vi "BRig_RT_panel_Laser1_v1,12.vi"(7 "input_setValues":bool, 9 "input_dataExp":u16[](array[numeric]), 11 "input_dataLC":u16[](array[numeric])) -> (1 "output_dataExp":u16[](array[numeric]), 3 "output_dataLC":u16[](array[numeric]))   [LabVIEW 2014]
panel:
  in  "LC_Wro_nRew2":u16
  in  "LC_Wro_nRew1":u16
  in  "LC_Rew_nRew2":u16
  in  "LC_Rew_nRew1":u16
  in  "LC_Sel_nRew2":u16
  in  "LC_Sel_nRew1":u16
  in  "LC_Cue2_nRew2":u16
  in  "LC_Cue2_nRew1":u16
  in  "LC_Cue_nRew2":u16
  in  "LC_Cue_nRew1":u16
  in  "LC_ENL2_nRew2":u16
  in  "LC_ENL2_nRew1":u16
  in  "LC_ENL_nRew2":u16
  in  "LC_ENL_nRew1":u16
  in  "LC_Cue2_PostR_Count":u16
  in  "LC_Cue2_PostR_delayOpt":bool
  in  "LC_Cue2_PostR_Probability":u16
  in  "LC_Cue2_PostR_Block":u16(slide) max=2 step=1 scale=0.0..2.0
  in  "LC_Cue2_PostR_OnOff":bool
  in  "LC_Cue2_PostR_Tdelay":u16
  in  "LC_ENL2_PostR_delayOpt":bool
  in  "LC_ENL2_PostR_Count":u16
  in  "LC_ENL2_PostR_Probability":u16 max=100 step=1
  in  "LC_ENL2_PostR_Block":u16(slide) max=2 step=1 scale=0.0..2.0
  in  "LC_ENL2_PostR_OnOff":bool
  in  "LC_ENL2_PostR_Tdelay":u16
  in  "LC_Cue2_PreR_Count":u16
  in  "LC_Cue2_First_Count":u16
  in  "LC_Cue2_PreR_delayOpt":bool
  in  "LC_ENL2_PreR_delayOpt":bool
  in  "LC_ENL2_PreR_Count":u16
  in  "LC_ENL2_First_Count":u16
  in  "LC_Cue2_First_delayOpt":bool
  in  "LC_ENL2_First_delayOpt":bool
  in  "LC_Cue2_PreR_Probability":u16
  in  "LC_Cue2_PreR_Block":u16(slide) max=2 step=1 scale=0.0..2.0
  in  "LC_Cue2_PreR_OnOff":bool
  in  "LC_Cue2_First_Probability":u16
  in  "LC_Cue2_First_Block":u16(slide) max=2 step=1 scale=0.0..2.0
  in  "LC_Cue2_First_OnOff":bool
  in  "LC_ENL2_PreR_Probability":u16 max=100 step=1
  in  "LC_ENL2_PreR_Block":u16(slide) max=2 step=1 scale=0.0..2.0
  in  "LC_ENL2_PreR_OnOff":bool
  in  "LC_ENL2_First_Probability":u16 max=100 step=1
  in  "LC_ENL2_First_Block":u16(slide) max=2 step=1 scale=0.0..2.0
  in  "LC_Cue2_PreR_Tdelay":u16
  in  "LC_ENL2_PreR_Tdelay":u16
  in  "LC_Cue2_First_Tdelay":u16
  in  "LC_ENL2_First_Tdelay":u16
  in  "LC_ENL2_First_OnOff":bool
  out "LaserPulseTrain":cluster{u16[], u16[]}(graph)
  in  "LED_baseline":bool
  in  "Laser_power_step":dbl
  in  "Laser_power_max":dbl
  in  "Laser_power_min":dbl
  in  "Laser_Tshutter":u16=2
  in  "Laser_Freq":u16=10
  in  "Laser_Tpeak":u16=2
  in  "Laser_T":u16
  in  "LC_Sel_PostR_Count":u16
  in  "LC_Sel_PostR_Probability":u16
  in  "LC_Sel_PostR_Block":u16(slide) max=2 step=1 scale=0.0..2.0
  in  "LC_Sel_PostR_OnOff":bool
  in  "LC_Sel_PostR_Tdelay":u16
  in  "LC_Cue_PostR_Count":u16
  in  "LC_Cue_PostR_delayOpt":bool
  in  "LC_Cue_PostR_Probability":u16
  in  "LC_Cue_PostR_Block":u16(slide) max=2 step=1 scale=0.0..2.0
  in  "LC_Cue_PostR_OnOff":bool
  in  "LC_Cue_PostR_Tdelay":u16
  in  "LC_ENL_PostR_delayOpt":bool
  in  "LC_ENL_PostR_Count":u16
  in  "LC_ENL_PostR_Probability":u16 max=100 step=1
  in  "LC_ENL_PostR_Block":u16(slide) max=2 step=1 scale=0.0..2.0
  in  "LC_ENL_PostR_OnOff":bool
  in  "LC_ENL_PostR_Tdelay":u16
  in  "LC_Sel_PreR_Count":u16
  in  "LC_Sel_First_Count":u16
  in  "LC_Sel_PreR_Probability":u16
  in  "LC_Sel_PreR_Block":u16(slide) max=2 step=1 scale=0.0..2.0
  in  "LC_Sel_PreR_OnOff":bool
  in  "LC_Sel_First_Probability":u16
  in  "LC_Sel_First_Block":u16(slide) max=2 step=1 scale=0.0..2.0
  in  "LC_Sel_First_OnOff":bool
  in  "LC_Sel_PreR_Tdelay":u16
  in  "LC_Sel_First_Tdelay":u16
  in  "LC_Cue_PreR_Count":u16
  in  "LC_Cue_First_Count":u16
  in  "LC_Cue_PreR_delayOpt":bool
  in  "LC_ENL_PreR_delayOpt":bool
  in  "LC_ENL_PreR_Count":u16
  in  "LC_ENL_First_Count":u16
  in  "LC_Cue_First_delayOpt":bool
  in  "LC_ENL_First_delayOpt":bool
  in  "LC_Wrong_Probability":u16
  in  "LC_Wrong_Trial":u16(slide) max=3 step=1 scale=0.0..3.0
  in  "LC_Wrong_Block":u16(slide) max=2 step=1 scale=0.0..2.0
  in  "LC_Wrong_OnOff":bool
  in  "LC_Reward_Probability":u16
  in  "LC_Reward_Trial":u16(slide) max=3 step=1 scale=0.0..3.0
  in  "LC_Reward_Block":u16(slide) max=2 step=1 scale=0.0..2.0
  in  "LC_Reward_OnOff":bool
  in  "LC_Cue_PreR_Probability":u16
  in  "LC_Cue_PreR_Block":u16(slide) max=2 step=1 scale=0.0..2.0
  in  "LC_Cue_PreR_OnOff":bool
  in  "LC_Cue_First_Probability":u16
  in  "LC_Cue_First_Block":u16(slide) max=2 step=1 scale=0.0..2.0
  in  "LC_Cue_First_OnOff":bool
  in  "LC_ENL_PreR_Probability":u16 max=100 step=1
  in  "LC_ENL_PreR_Block":u16(slide) max=2 step=1 scale=0.0..2.0
  in  "LC_ENL_PreR_OnOff":bool
  in  "LC_ENL_First_Probability":u16 max=100 step=1
  in  "LC_ENL_First_Block":u16(slide) max=2 step=1 scale=0.0..2.0
  in  "LC_Wrong_Tdelay":u16
  in  "LC_Cue_PreR_Tdelay":u16
  in  "LC_ENL_PreR_Tdelay":u16
  in  "LC_Reward_Tdelay":u16
  in  "LC_Cue_First_Tdelay":u16
  in  "LC_ENL_First_Tdelay":u16
  in  "LC_ENL_First_OnOff":bool
  # "Laser1 Control\n                               On/Off      Block        Probability [%]   Delay [ms]                              Count"
  # "On/Off      Block        Probability [%]   Delay [ms]                              Count"
  # "Enforced\nNonLick"
  # "Enforced\nNonLick\n     2"
  # "from end"
  # "from end"
  # "First\nTrial"
  # "First\nTrial"
  # "from start"
  # "from start"
  # "from end"
  # "from end"
  # "PreReward\nTrials"
  # "PreReward\nTrials"
  # "from start"
  # "from start"
  # "from end"
  # "from end"
  # "PostReward\nTrials"
  # "PostReward\nTrials"
  # "from start"
  # "from start"
  # "PostReward Option - Trigger after [X1] or [X2] reward\n                                        (0 = ignore this option)"
  # "PostReward Option - Trigger after [X1] or [X2] reward\n                                        (0 = ignore this option)"
  # "Cue"
  # "Cue\n  2"
  # "from end"
  # "from end"
  # "First\nTrial"
  # "First\nTrial"
  # "from start"
  # "from start"
  # "from end"
  # "from end"
  # "PreReward\nTrials"
  # "PreReward\nTrials"
  # "from start"
  # "from start"
  # "from end"
  # "from end"
  # "PostReward\nTrials"
  # "PostReward\nTrials"
  # "from start"
  # "from start"
  # "PostReward Option - Trigger after [X1] or [X2] reward\n                                        (0 = ignore this option)"
  # "PostReward Option - Trigger after [X1] or [X2] reward\n                                        (0 = ignore this option)"
  # "Selection"
  # "from start"
  # "First\nTrial"
  # "from start"
  # "PreReward\nTrials"
  # "from start"
  # "PostReward\nTrials"
  # "PostReward Option - Trigger after [X1] or [X2] reward\n                                        (0 = ignore this option)"
  # "Laser1 Parameters"
  # "Laser1 Response\n           On/Off      Block           Trial     Probability %  Delay [ms]"
  # "Frequency\n[Hz]"
  # "Selection\nReward"
  # "Timing [ms]\n Duration     Peak Width   Shutter"
  # "Trigger after [X1] or [X2] reward\n(0 = ignore this option)"
  # "Laser Power [V]\nMin          Max              Step"
  # "Selection\nWrong"
  # "Trigger after [X1] or [X2] reward\n(0 = ignore this option)"
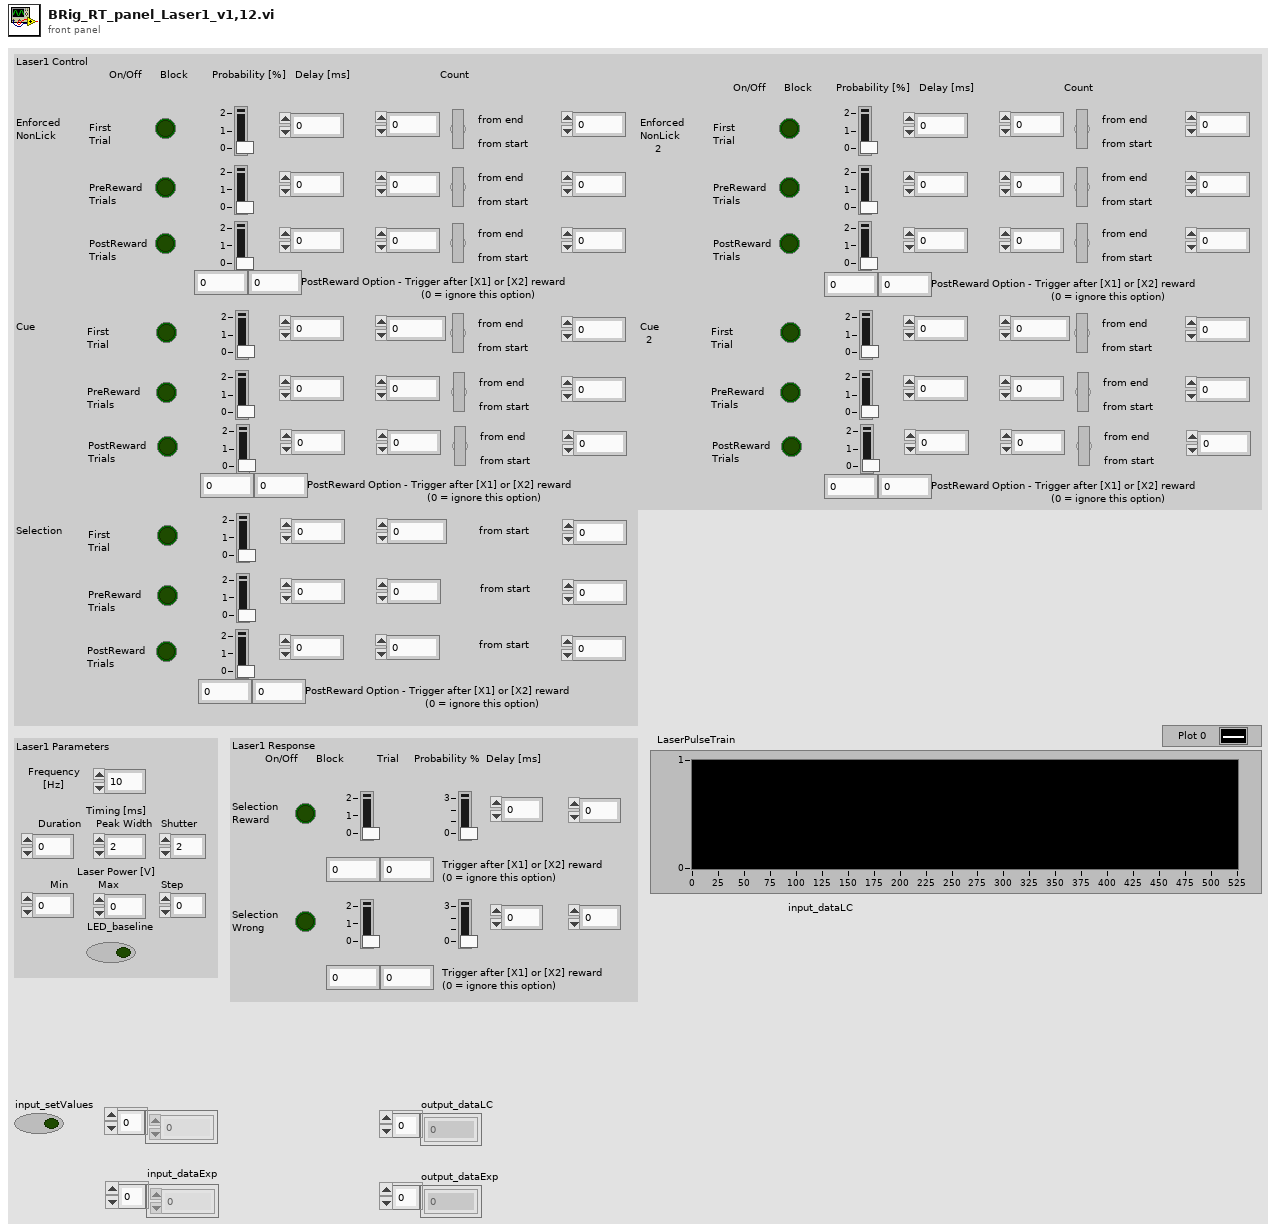
[diagram p1: front panel]
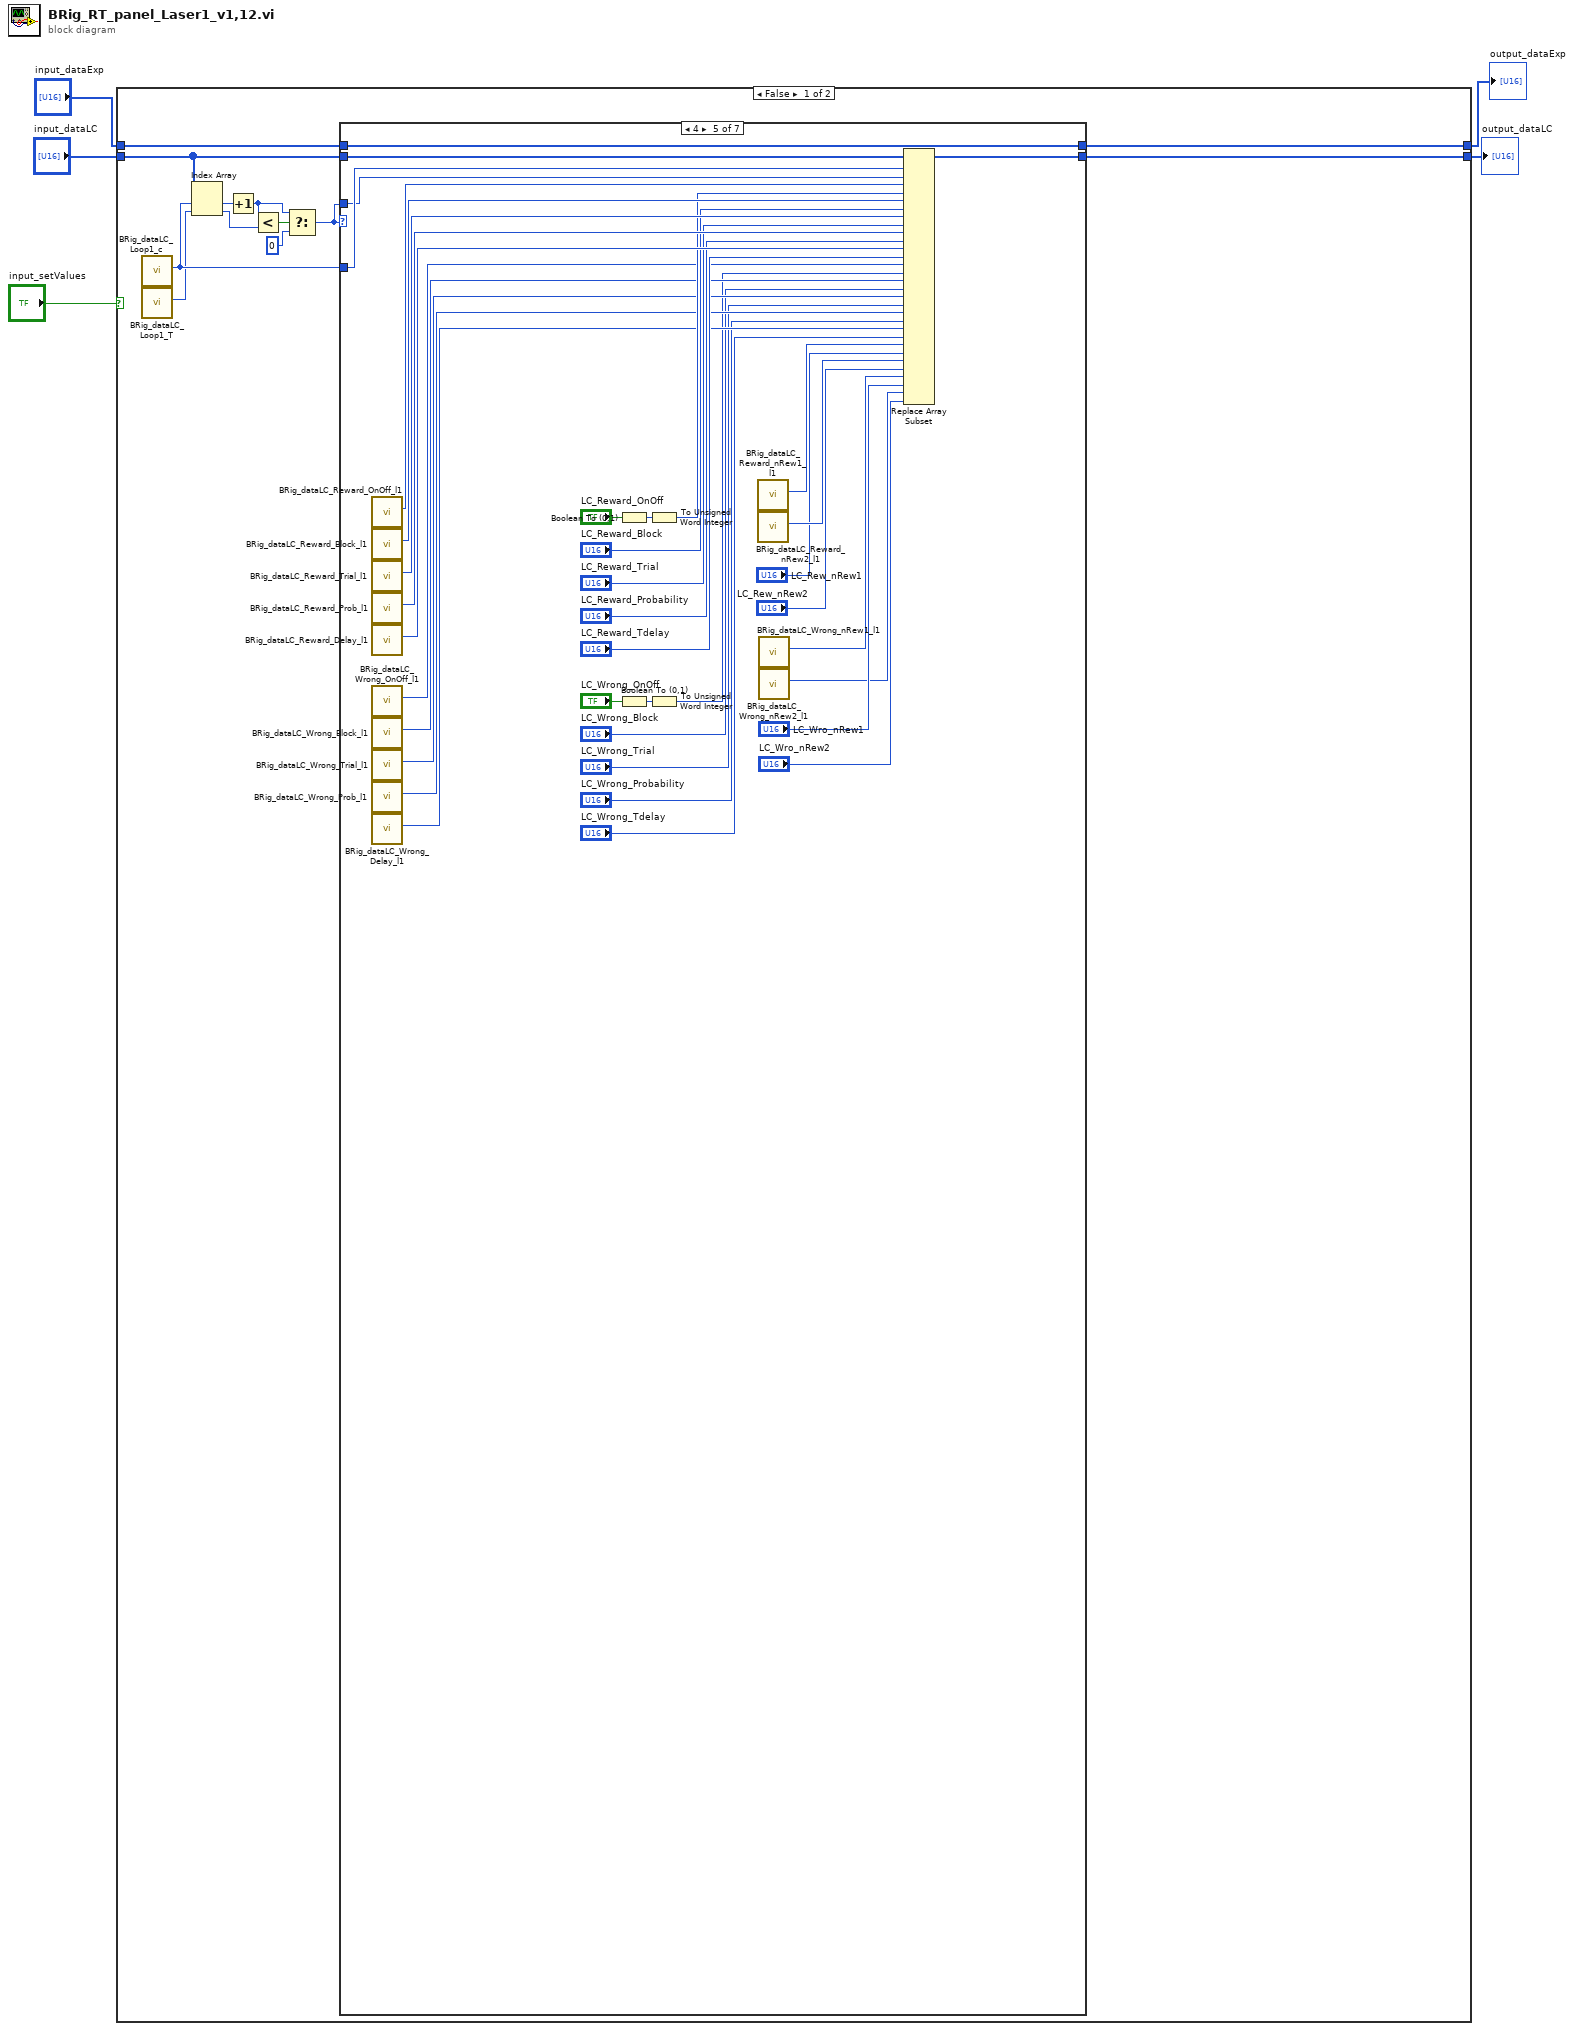
[diagram p0: block diagram]
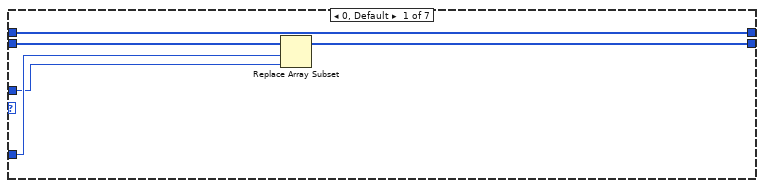
[diagram p2: hidden frame]
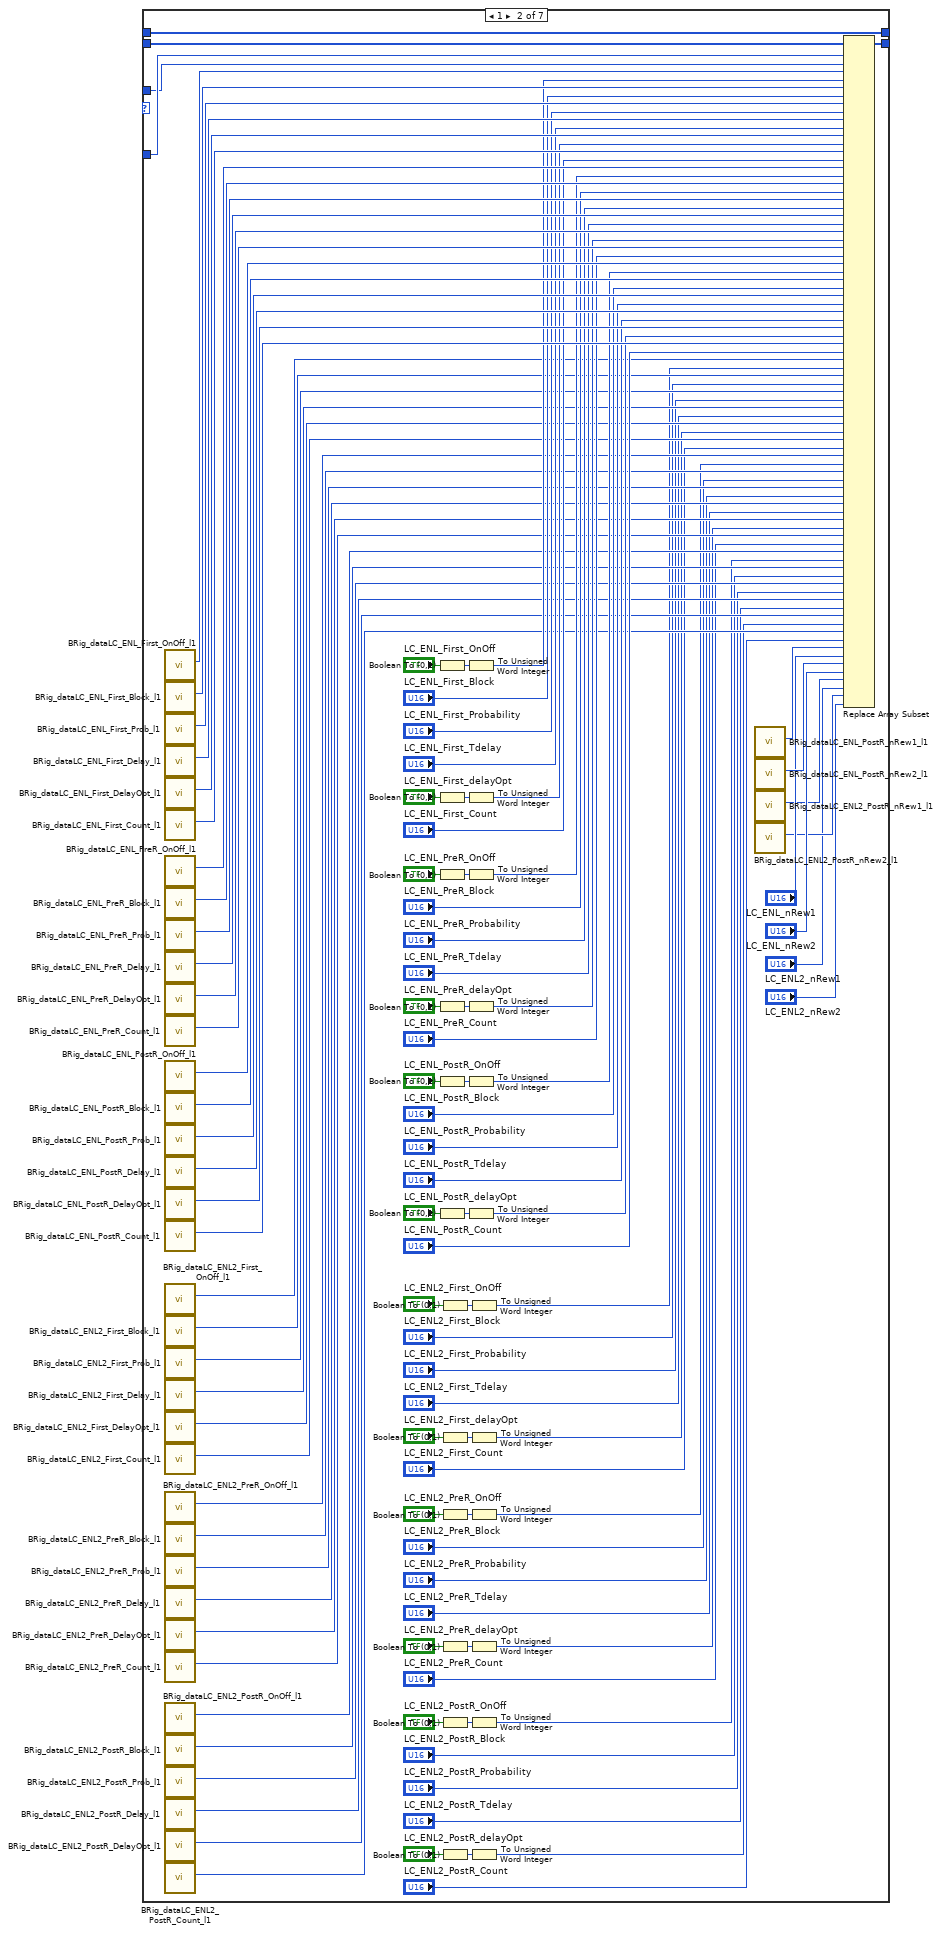
[diagram p3: hidden frame]
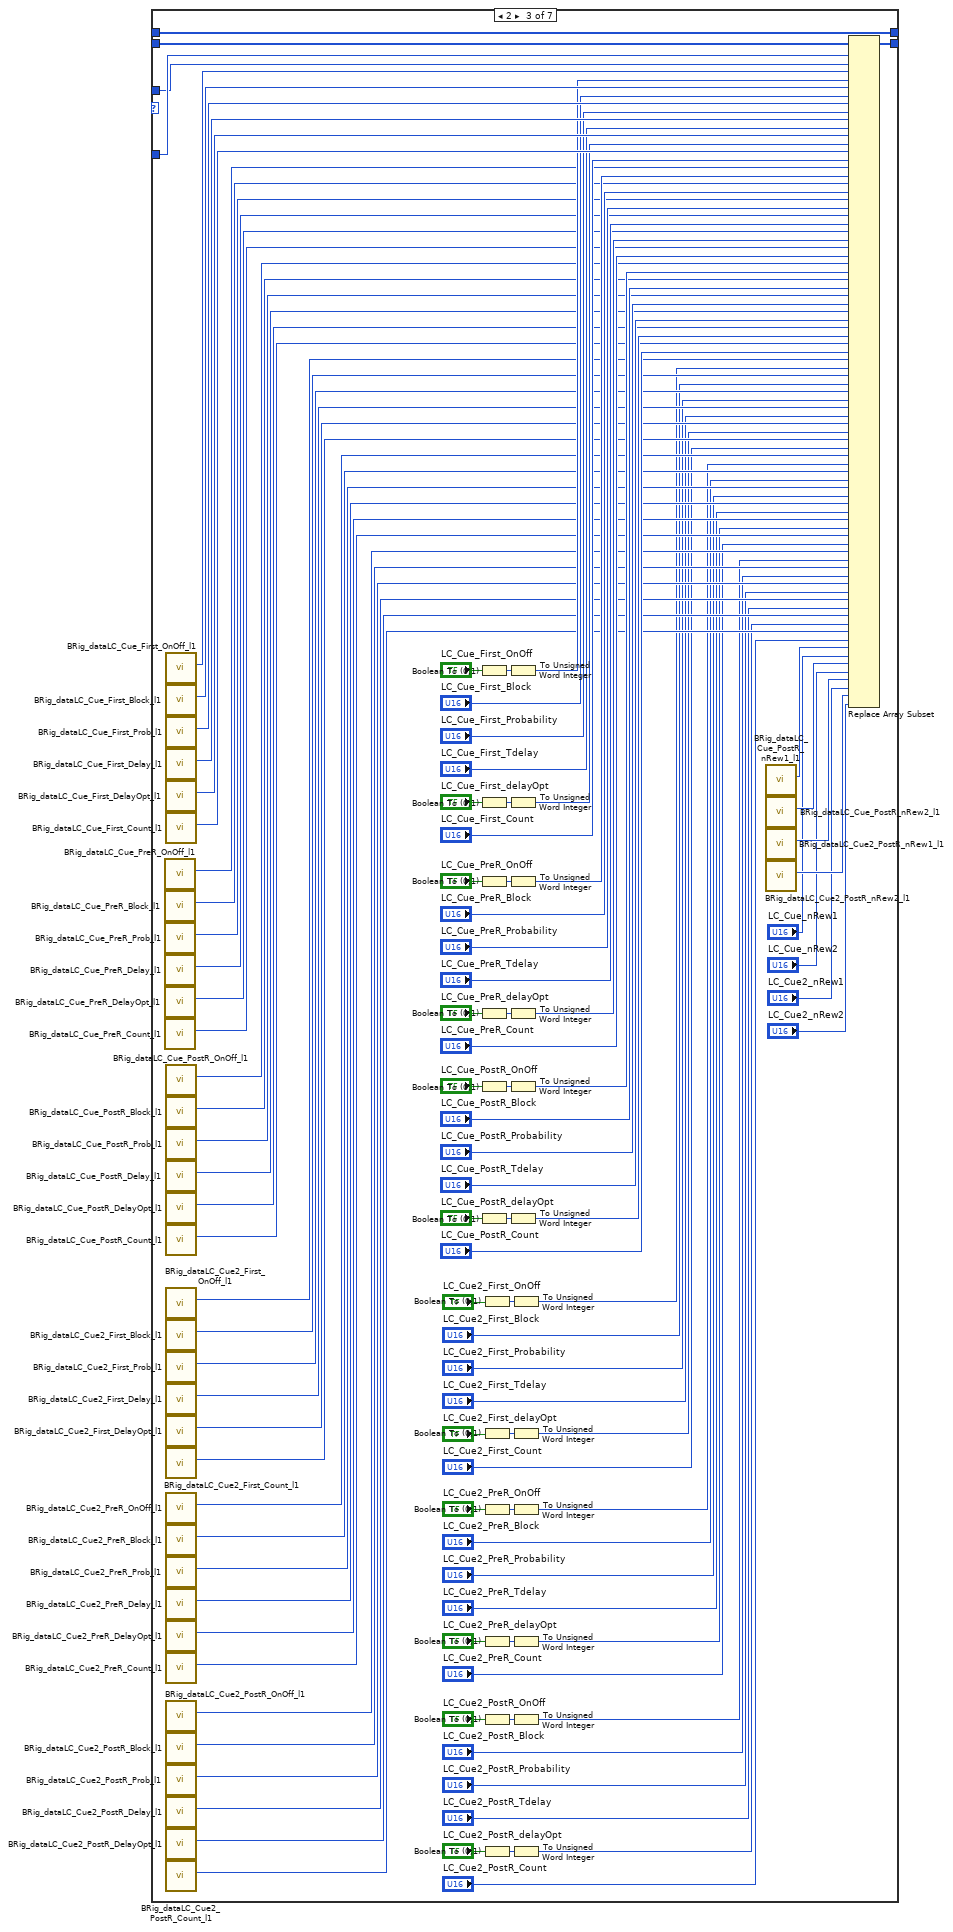
[diagram p4: hidden frame]
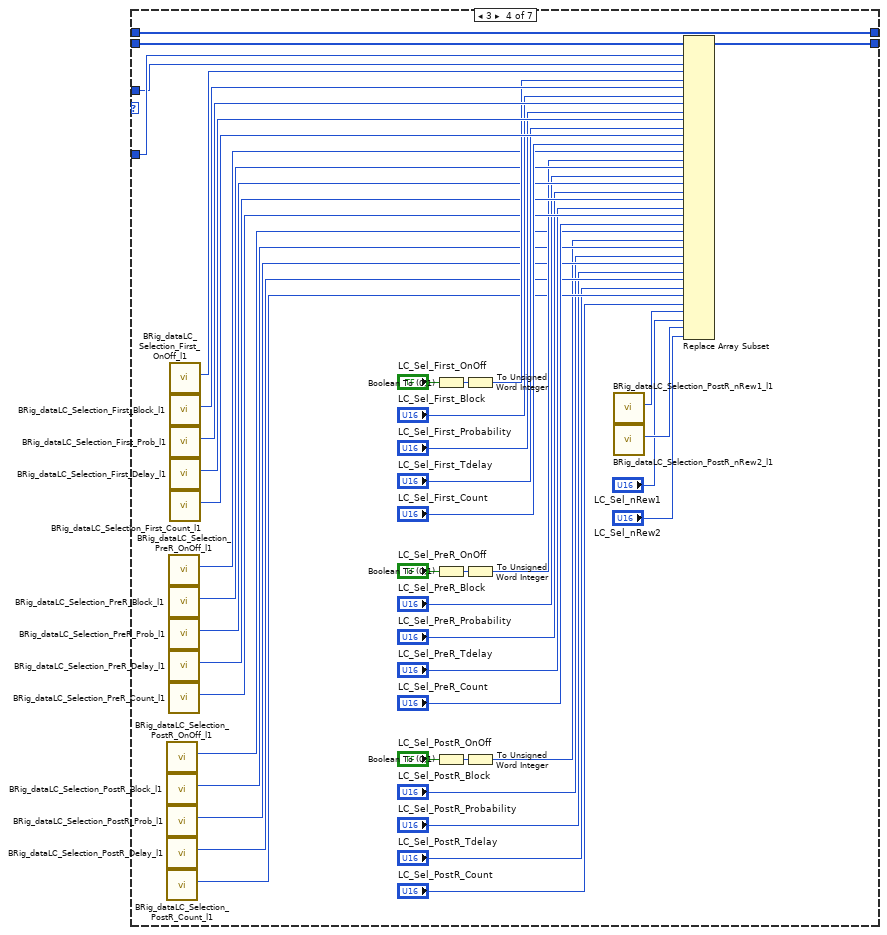
[diagram p5: hidden frame]
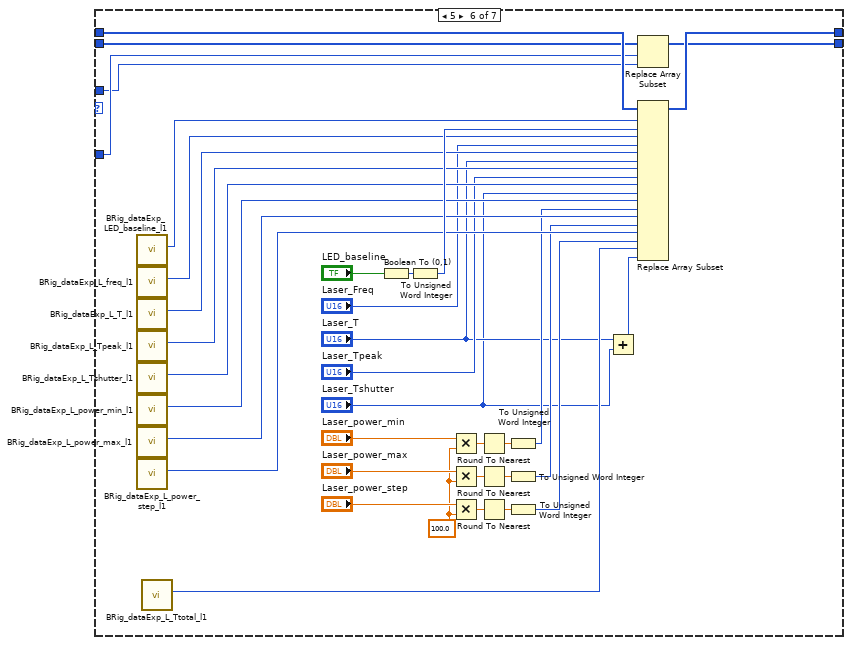
[diagram p6: hidden frame]
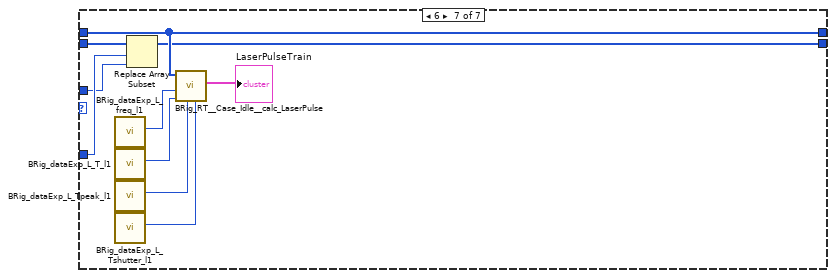
[diagram p7: hidden frame]
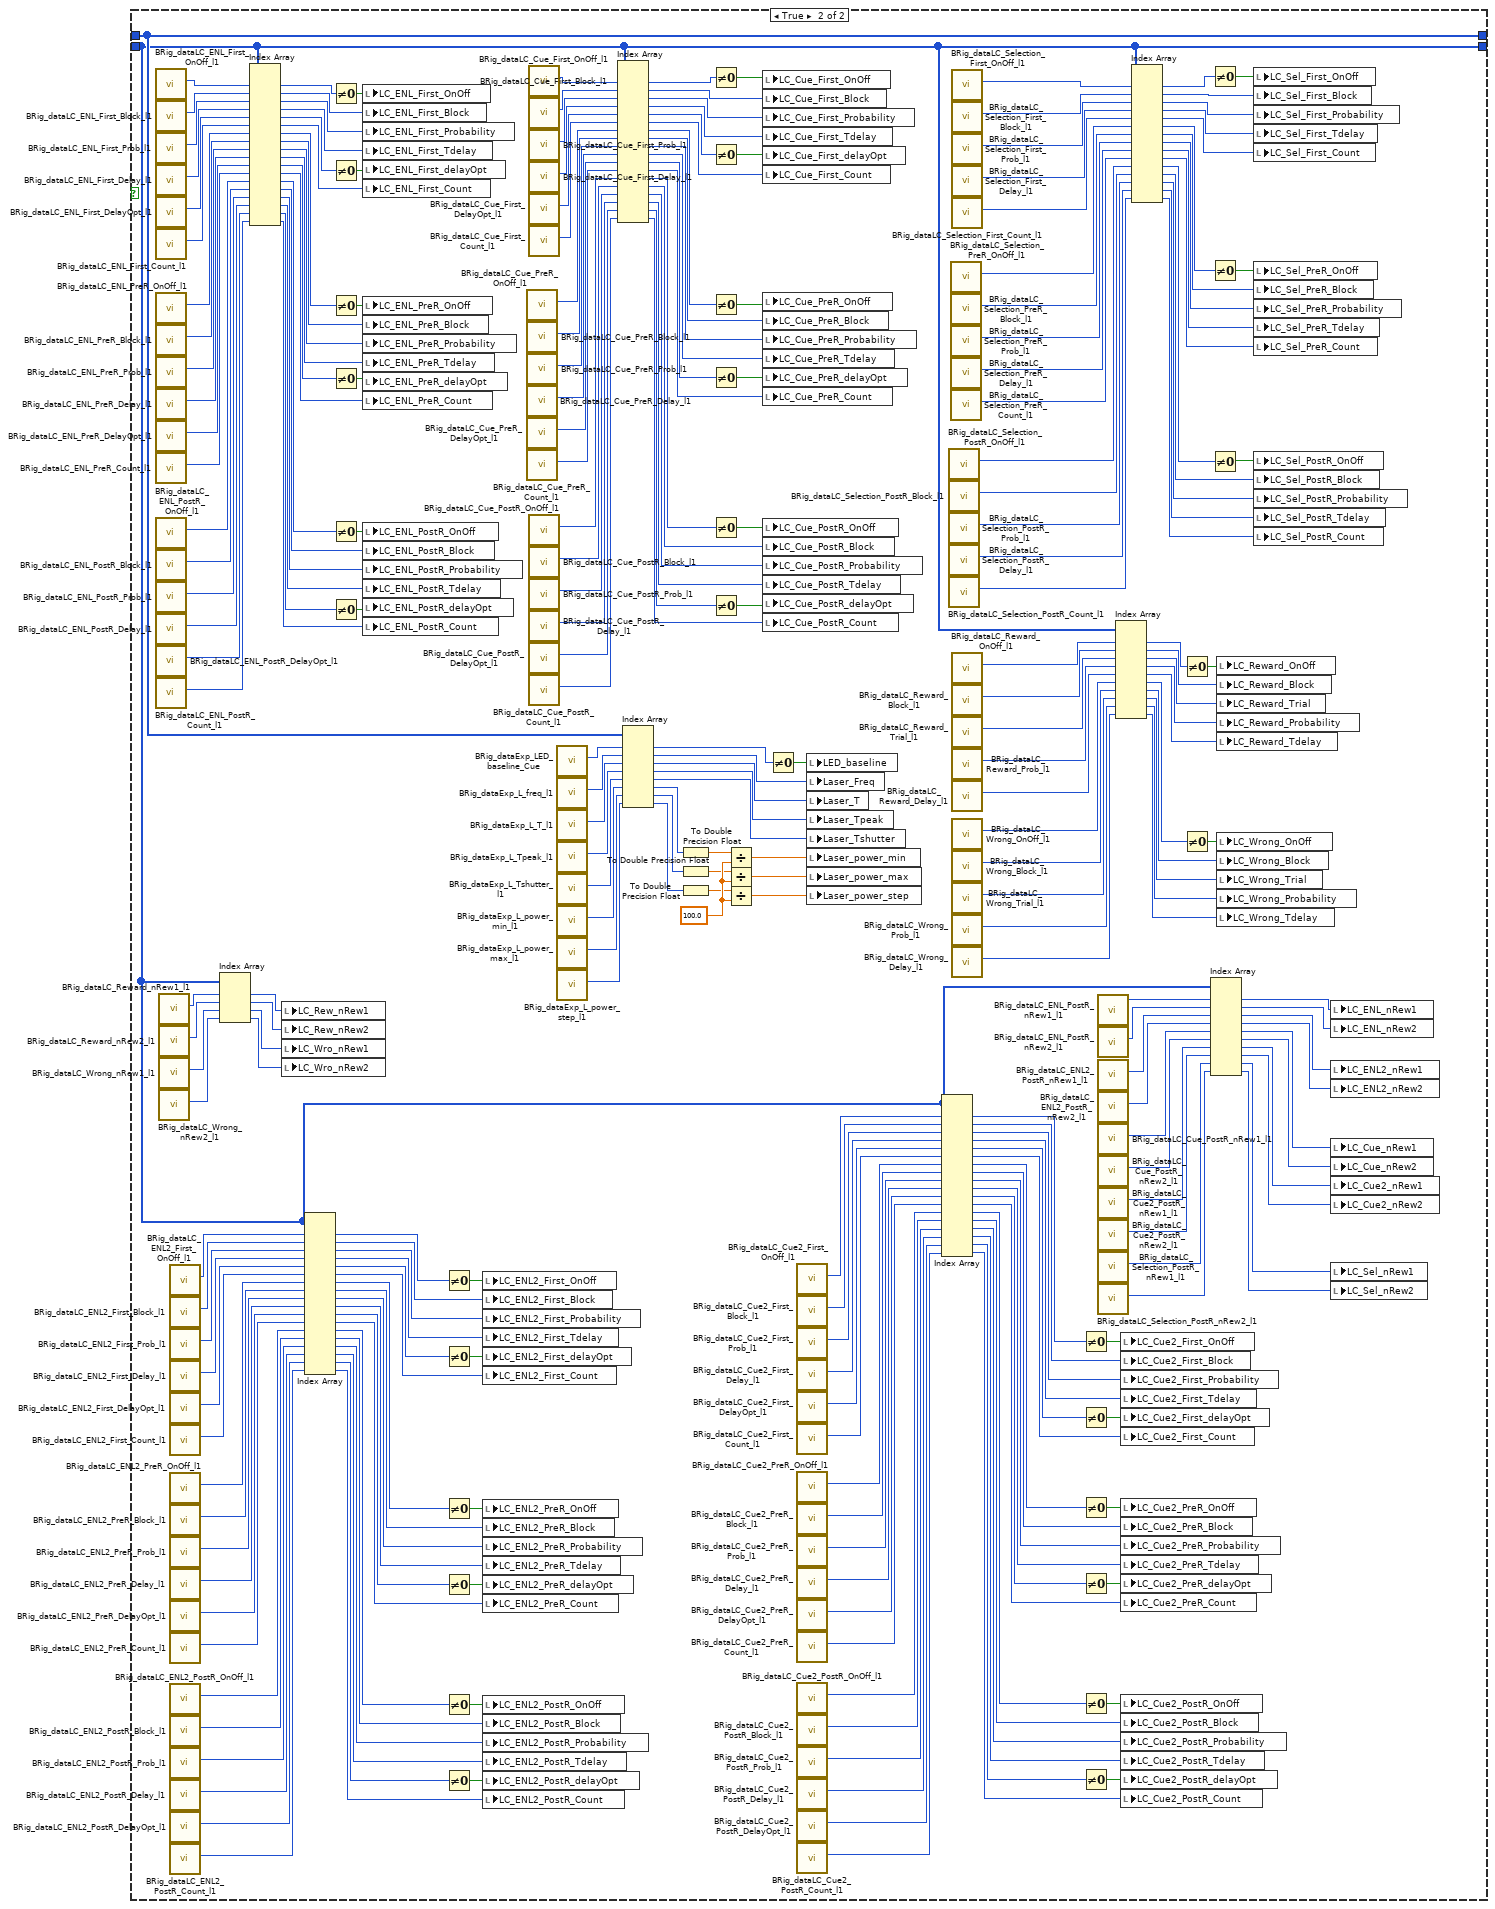
[diagram p8: hidden frame]
diagram:
  n1 = case shown="False" "input_setValues" {
    tunnel: "input_dataLC" -> [w17 w377]
    tunnel: [w11 w377] -> w4
    tunnel: "input_dataExp" -> [w7 w394]
    tunnel: [w6 w394] -> w1
    frame False {
      n2 = call "BRig_dataLC_Loop1_c.vi"() -> ("output_Loop1_c"=w10:i32)  [unwired: 11 in]
      n3 = call "BRig_dataLC_Loop1_T.vi"() -> ("output_Loop1_T"=w9:i32)  [unwired: 11 in]
      n4 = Index Array(array=w17, index #1=w10, index #2=w9) -> (element #1=w16:u16, element #2=w15:u16)
      n5 = Increment(x=w16) -> (x+1=w12:u16)
      n6 = Less?(x=w12, y=w15) -> (x < y?=w14:bool)
      n7 = Select(t=w12, s=w14, f=u16 0) -> (s? t:f=w8:u16)
      n8 = case shown="4" w8 {
        tunnel: w17 -> [w22 w131 w240 w285 w322 w327 w366]
        tunnel: w10 -> [w20 w81 w202 w247 w296 w325 w364]
        tunnel: w8 -> [w19 w80 w201 w246 w295 w324 w363]
        tunnel: [w21 w124 w239 w284 w321 w326 w365] -> w11
        tunnel: w7 -> [w18 w79 w188 w245 w294 w329 w368]
        tunnel: [w18 w79 w188 w245 w294 w328 w368] -> w6
        frame 0, Default {
          n9 = Replace Array Subset(array=w22, new element=w19, index=w20) -> (w21:u16[])
        }
        frame 1 {
          n10 = call "BRig_dataLC_ENL_First_OnOff_l1.vi"() -> ("output_ENL_First_OnOff"=w130:i32)  [unwired: 11 in]
          n11 = call "BRig_dataLC_ENL_First_Block_l1.vi"() -> ("output_ENL_First_Block"=w129:i32)  [unwired: 11 in]
          n12 = call "BRig_dataLC_ENL_First_Prob_l1.vi"() -> ("output_ENL_First_Prob"=w128:i32)  [unwired: 11 in]
          n13 = call "BRig_dataLC_ENL_First_Delay_l1.vi"() -> ("output_ENL_First_Delay"=w127:i32)  [unwired: 11 in]
          n14 = call "BRig_dataLC_ENL_First_DelayOpt_l1.vi"() -> ("output_ENL_First_DelayOpt"=w126:i32)  [unwired: 11 in]
          n15 = call "BRig_dataLC_ENL_First_Count_l1.vi"() -> ("output_ENL_First_Count"=w125:i32)  [unwired: 11 in]
          n16 = call "BRig_dataLC_ENL_PreR_OnOff_l1.vi"() -> ("output_ENL_PreR_OnOff"=w123:i32)  [unwired: 11 in]
          n17 = call "BRig_dataLC_ENL_PreR_Block_l1.vi"() -> ("output_ENL_PreR_Block"=w122:i32)  [unwired: 11 in]
          n18 = call "BRig_dataLC_ENL_PreR_Prob_l1.vi"() -> ("output_ENL_PreR_Prob"=w121:i32)  [unwired: 11 in]
          n19 = call "BRig_dataLC_ENL_PreR_Delay_l1.vi"() -> ("output_ENL_PreR_Delay"=w120:i32)  [unwired: 11 in]
          n20 = call "BRig_dataLC_ENL_PreR_DelayOpt_l1.vi"() -> ("output_ENL_PreR_DelayOpt"=w119:i32)  [unwired: 11 in]
          n21 = call "BRig_dataLC_ENL_PreR_Count_l1.vi"() -> ("output_ENL_PreR_Count"=w118:i32)  [unwired: 11 in]
          n22 = call "BRig_dataLC_ENL_PostR_OnOff_l1.vi"() -> ("output_ENL_PostR_OnOff"=w117:i32)  [unwired: 11 in]
          n23 = call "BRig_dataLC_ENL_PostR_Block_l1.vi"() -> ("output_ENL_PostR_Block"=w116:i32)  [unwired: 11 in]
          n24 = call "BRig_dataLC_ENL_PostR_Prob_l1.vi"() -> ("output_ENL_PostR_Prob"=w115:i32)  [unwired: 11 in]
          n25 = call "BRig_dataLC_ENL_PostR_Delay_l1.vi"() -> ("output_ENL_PostR_Delay"=w114:i32)  [unwired: 11 in]
          n26 = call "BRig_dataLC_ENL_PostR_DelayOpt_l1.vi"() -> ("output_ENL_PostR_DelayOpt"=w113:i32)  [unwired: 11 in]
          n27 = call "BRig_dataLC_ENL_PostR_Count_l1.vi"() -> ("output_ENL_PostR_Count"=w112:i32)  [unwired: 11 in]
          n28 = call "BRig_dataLC_ENL2_First_OnOff_l1.vi"() -> ("output_ENL2_First_OnOff"=w78:i32)  [unwired: 11 in]
          n29 = call "BRig_dataLC_ENL2_First_Block_l1.vi"() -> ("output_ENL2_First_Block"=w77:i32)  [unwired: 11 in]
          n30 = call "BRig_dataLC_ENL2_First_Prob_l1.vi"() -> ("output_ENL2_First_Prob"=w76:i32)  [unwired: 11 in]
          n31 = call "BRig_dataLC_ENL2_First_Delay_l1.vi"() -> ("output_ENL2_First_Delay"=w75:i32)  [unwired: 11 in]
          n32 = call "BRig_dataLC_ENL2_First_DelayOpt_l1.vi"() -> ("output_ENL2_First_DelayOpt"=w74:i32)  [unwired: 11 in]
          n33 = call "BRig_dataLC_ENL2_First_Count_l1.vi"() -> ("output_ENL2_First_Count"=w73:i32)  [unwired: 11 in]
          n34 = call "BRig_dataLC_ENL2_PreR_OnOff_l1.vi"() -> ("output_ENL2_PreR_OnOff"=w72:i32)  [unwired: 11 in]
          n35 = call "BRig_dataLC_ENL2_PreR_Block_l1.vi"() -> ("output_ENL2_PreR_Block"=w71:i32)  [unwired: 11 in]
          n36 = call "BRig_dataLC_ENL2_PreR_Prob_l1.vi"() -> ("output_ENL2_PreR_Prob"=w70:i32)  [unwired: 11 in]
          n37 = call "BRig_dataLC_ENL2_PreR_Delay_l1.vi"() -> ("output_ENL2_PreR_Delay"=w69:i32)  [unwired: 11 in]
          n38 = call "BRig_dataLC_ENL2_PreR_DelayOpt_l1.vi"() -> ("output_ENL2_PreR_DelayOpt"=w68:i32)  [unwired: 11 in]
          n39 = call "BRig_dataLC_ENL2_PreR_Count_l1.vi"() -> ("output_ENL2_PreR_Count"=w67:i32)  [unwired: 11 in]
          n40 = call "BRig_dataLC_ENL2_PostR_OnOff_l1.vi"() -> ("output_ENL2_PostR_OnOff"=w66:i32)  [unwired: 11 in]
          n41 = call "BRig_dataLC_ENL2_PostR_Block_l1.vi"() -> ("output_ENL2_PostR_Block"=w65:i32)  [unwired: 11 in]
          n42 = call "BRig_dataLC_ENL2_PostR_Prob_l1.vi"() -> ("output_ENL2_PostR_Prob"=w64:i32)  [unwired: 11 in]
          n43 = call "BRig_dataLC_ENL2_PostR_Delay_l1.vi"() -> ("output_ENL2_PostR_Delay"=w63:i32)  [unwired: 11 in]
          n44 = call "BRig_dataLC_ENL2_PostR_DelayOpt_l1.vi"() -> ("output_ENL2_PostR_DelayOpt"=w62:i32)  [unwired: 11 in]
          n45 = call "BRig_dataLC_ENL2_PostR_Count_l1.vi"() -> ("output_ENL2_PostR_Count"=w61:i32)  [unwired: 11 in]
          n46 = Boolean To (0,1)(Boolean="LC_ENL_First_OnOff") -> (0, 1=w110:i16)
          n47 = Boolean To (0,1)(Boolean="LC_ENL_First_delayOpt") -> (0, 1=w109:i16)
          n48 = Boolean To (0,1)(Boolean="LC_ENL_PreR_OnOff") -> (0, 1=w107:i16)
          n49 = Boolean To (0,1)(Boolean="LC_ENL_PreR_delayOpt") -> (0, 1=w105:i16)
          n50 = Boolean To (0,1)(Boolean="LC_ENL_PostR_OnOff") -> (0, 1=w103:i16)
          n51 = Boolean To (0,1)(Boolean="LC_ENL_PostR_delayOpt") -> (0, 1=w101:i16)
          n52 = Boolean To (0,1)(Boolean="LC_ENL2_First_OnOff") -> (0, 1=w51:i16)
          n53 = Boolean To (0,1)(Boolean="LC_ENL2_First_delayOpt") -> (0, 1=w50:i16)
          n54 = Boolean To (0,1)(Boolean="LC_ENL2_PreR_OnOff") -> (0, 1=w49:i16)
          n55 = Boolean To (0,1)(Boolean="LC_ENL2_PreR_delayOpt") -> (0, 1=w47:i16)
          n56 = Boolean To (0,1)(Boolean="LC_ENL2_PostR_OnOff") -> (0, 1=w39:i16)
          n57 = Boolean To (0,1)(Boolean="LC_ENL2_PostR_delayOpt") -> (0, 1=w37:i16)
          n58 = To Unsigned Word Integer(number=w110) -> (unsigned 16bit integer=w99:u16)
          n59 = To Unsigned Word Integer(number=w109) -> (unsigned 16bit integer=w95:u16)
          n60 = To Unsigned Word Integer(number=w107) -> (unsigned 16bit integer=w93:u16)
          n61 = To Unsigned Word Integer(number=w105) -> (unsigned 16bit integer=w89:u16)
          n62 = To Unsigned Word Integer(number=w103) -> (unsigned 16bit integer=w87:u16)
          n63 = To Unsigned Word Integer(number=w101) -> (unsigned 16bit integer=w83:u16)
          n64 = To Unsigned Word Integer(number=w51) -> (unsigned 16bit integer=w58:u16)
          n65 = To Unsigned Word Integer(number=w50) -> (unsigned 16bit integer=w54:u16)
          n66 = To Unsigned Word Integer(number=w49) -> (unsigned 16bit integer=w52:u16)
          n67 = To Unsigned Word Integer(number=w47) -> (unsigned 16bit integer=w42:u16)
          n68 = To Unsigned Word Integer(number=w39) -> (unsigned 16bit integer=w40:u16)
          n69 = To Unsigned Word Integer(number=w37) -> (unsigned 16bit integer=w32:u16)
          n70 = call "BRig_dataLC_ENL_PostR_nRew1_l1.vi"() -> ("output_ENL_PostR_nRew1_l1"=w30:i32)  [unwired: 11 in]
          n71 = call "BRig_dataLC_ENL_PostR_nRew2_l1.vi"() -> ("output_ENL_PostR_nRew2_l1"=w29:i32)  [unwired: 11 in]
          n72 = call "BRig_dataLC_ENL2_PostR_nRew1_l1.vi"() -> ("output_ENL2_PostR_nRew1_l1"=w26:i32)  [unwired: 11 in]
          n73 = call "BRig_dataLC_ENL2_PostR_nRew2_l1.vi"() -> ("output_ENL2_PostR_nRew2_l1"=w25:i32)  [unwired: 11 in]
          n74 = Replace Array Subset(array=w131, new element #1=w80, index #1=w81, new element #2=w99, index #2=w130, new element #3="LC_ENL_First_Block", index #3=w129, new element #4="LC_ENL_First_Probability", index #4=w128, new element #5="LC_ENL_First_Tdelay", index #5=w127, new element #6=w95, index #6=w126, new element #7="LC_ENL_First_Count", index #7=w125, new element #8=w93, index #8=w123, new element #9="LC_ENL_PreR_Block", index #9=w122, new element #10="LC_ENL_PreR_Probability", index #10=w121, new element #11="LC_ENL_PreR_Tdelay", index #11=w120, new element #12=w89, index #12=w119, new element #13="LC_ENL_PreR_Count", index #13=w118, new element #14=w87, index #14=w117, new element #15="LC_ENL_PostR_Block", index #15=w116, new element #16="LC_ENL_PostR_Probability", index #16=w115, new element #17="LC_ENL_PostR_Tdelay", index #17=w114, new element #18=w83, index #18=w113, new element #19="LC_ENL_PostR_Count", index #19=w112, new element #20=w58, index #20=w78, new element #21="LC_ENL2_First_Block", index #21=w77, new element #22="LC_ENL2_First_Probability", index #22=w76, new element #23="LC_ENL2_First_Tdelay", index #23=w75, new element #24=w54, index #24=w74, new element #25="LC_ENL2_First_Count", index #25=w73, new element #26=w52, index #26=w72, new element #27="LC_ENL2_PreR_Block", index #27=w71, new element #28="LC_ENL2_PreR_Probability", index #28=w70, new element #29="LC_ENL2_PreR_Tdelay", index #29=w69, new element #30=w42, index #30=w68, new element #31="LC_ENL2_PreR_Count", index #31=w67, new element #32=w40, index #32=w66, new element #33="LC_ENL2_PostR_Block", index #33=w65, new element #34="LC_ENL2_PostR_Probability", index #34=w64, new element #35="LC_ENL2_PostR_Tdelay", index #35=w63, new element #36=w32, index #36=w62, new element #37="LC_ENL2_PostR_Count", index #37=w61, new element #38="LC_ENL_nRew1", index #38=w30, new element #39="LC_ENL_nRew2", index #39=w29, new element #40="LC_ENL2_nRew1", index #40=w26, new element #41="LC_ENL2_nRew2", index #41=w25) -> (w124:u16[])
        }
        frame 2 {
          n75 = call "BRig_dataLC_Cue_PreR_OnOff_l1.vi"() -> ("output_Cue_PreR_OnOff"=w198:i32)  [unwired: 11 in]
          n76 = call "BRig_dataLC_Cue_PreR_Block_l1.vi"() -> ("output_Cue_PreR_Block"=w197:i32)  [unwired: 11 in]
          n77 = call "BRig_dataLC_Cue_PreR_Prob_l1.vi"() -> ("output_Cue_PreR_Prob"=w196:i32)  [unwired: 11 in]
          n78 = call "BRig_dataLC_Cue_PreR_Delay_l1.vi"() -> ("output_Cue_PreR_Delay"=w195:i32)  [unwired: 11 in]
          n79 = call "BRig_dataLC_Cue_PreR_DelayOpt_l1.vi"() -> ("output_Cue_PreR_DelayOpt"=w194:i32)  [unwired: 11 in]
          n80 = call "BRig_dataLC_Cue_PreR_Count_l1.vi"() -> ("output_Cue_PreR_Count"=w199:i32)  [unwired: 11 in]
          n81 = call "BRig_dataLC_Cue_First_OnOff_l1.vi"() -> ("output_Cue_First_OnOff"=w238:i32)  [unwired: 11 in]
          n82 = call "BRig_dataLC_Cue_First_Block_l1.vi"() -> ("output_Cue_First_Block"=w237:i32)  [unwired: 11 in]
          n83 = call "BRig_dataLC_Cue_First_Prob_l1.vi"() -> ("output_Cue_First_Prob"=w236:i32)  [unwired: 11 in]
          n84 = call "BRig_dataLC_Cue_First_Delay_l1.vi"() -> ("output_Cue_First_Delay"=w235:i32)  [unwired: 11 in]
          n85 = call "BRig_dataLC_Cue_First_DelayOpt_l1.vi"() -> ("output_Cue_First_DelayOpt"=w234:i32)  [unwired: 11 in]
          n86 = call "BRig_dataLC_Cue_First_Count_l1.vi"() -> ("output_Cue_First_Count"=w233:i32)  [unwired: 11 in]
          n87 = call "BRig_dataLC_Cue_PostR_OnOff_l1.vi"() -> ("output_Cue_PostR_OnOff"=w200:i32)  [unwired: 11 in]
          n88 = call "BRig_dataLC_Cue_PostR_Block_l1.vi"() -> ("output_Cue_PostR_Block"=w193:i32)  [unwired: 11 in]
          n89 = call "BRig_dataLC_Cue_PostR_Prob_l1.vi"() -> ("output_Cue_PostR_Prob"=w192:i32)  [unwired: 11 in]
          n90 = call "BRig_dataLC_Cue_PostR_Delay_l1.vi"() -> ("output_Cue_PostR_Delay"=w191:i32)  [unwired: 11 in]
          n91 = call "BRig_dataLC_Cue_PostR_DelayOpt_l1.vi"() -> ("output_Cue_PostR_DelayOpt"=w190:i32)  [unwired: 11 in]
          n92 = call "BRig_dataLC_Cue_PostR_Count_l1.vi"() -> ("output_Cue_PostR_Count"=w189:i32)  [unwired: 11 in]
          n93 = call "BRig_dataLC_Cue2_First_OnOff_l1.vi"() -> ("output_Cue2_First_OnOff"=w187:i32)  [unwired: 11 in]
          n94 = call "BRig_dataLC_Cue2_First_Block_l1.vi"() -> ("output_Cue2_First_Block"=w186:i32)  [unwired: 11 in]
          n95 = call "BRig_dataLC_Cue2_First_Prob_l1.vi"() -> ("output_Cue2_First_Prob"=w185:i32)  [unwired: 11 in]
          n96 = call "BRig_dataLC_Cue2_First_Delay_l1.vi"() -> ("output_Cue2_First_Delay"=w184:i32)  [unwired: 11 in]
          n97 = call "BRig_dataLC_Cue2_First_DelayOpt_l1.vi"() -> ("output_Cue2_First_DelayOpt"=w183:i32)  [unwired: 11 in]
          n98 = call "BRig_dataLC_Cue2_First_Count_l1.vi"() -> ("output_Cue2_First_Count"=w182:i32)  [unwired: 11 in]
          n99 = call "BRig_dataLC_Cue2_PreR_OnOff_l1.vi"() -> ("output_Cue2_PreR_OnOff"=w181:i32)  [unwired: 11 in]
          n100 = call "BRig_dataLC_Cue2_PreR_Block_l1.vi"() -> ("output_Cue2_PreR_Block"=w180:i32)  [unwired: 11 in]
          n101 = call "BRig_dataLC_Cue2_PreR_Prob_l1.vi"() -> ("output_Cue2_PreR_Prob"=w179:i32)  [unwired: 11 in]
          n102 = call "BRig_dataLC_Cue2_PreR_Delay_l1.vi"() -> ("output_Cue2_PreR_Delay"=w178:i32)  [unwired: 11 in]
          n103 = call "BRig_dataLC_Cue2_PreR_DelayOpt_l1.vi"() -> ("output_Cue2_PreR_DelayOpt"=w177:i32)  [unwired: 11 in]
          n104 = call "BRig_dataLC_Cue2_PreR_Count_l1.vi"() -> ("output_Cue2_PreR_Count"=w176:i32)  [unwired: 11 in]
          n105 = call "BRig_dataLC_Cue2_PostR_OnOff_l1.vi"() -> ("output_Cue2_PostR_OnOff"=w175:i32)  [unwired: 11 in]
          n106 = call "BRig_dataLC_Cue2_PostR_Block_l1.vi"() -> ("output_Cue2_PostR_Block"=w174:i32)  [unwired: 11 in]
          n107 = call "BRig_dataLC_Cue2_PostR_Prob_l1.vi"() -> ("output_Cue2_PostR_Prob"=w173:i32)  [unwired: 11 in]
          n108 = call "BRig_dataLC_Cue2_PostR_Delay_l1.vi"() -> ("output_Cue2_PostR_Delay"=w172:i32)  [unwired: 11 in]
          n109 = call "BRig_dataLC_Cue2_PostR_DelayOpt_l1.vi"() -> ("output_Cue2_PostR_DelayOpt"=w171:i32)  [unwired: 11 in]
          n110 = call "BRig_dataLC_Cue2_PostR_Count_l1.vi"() -> ("output_Cue2_PostR_Count"=w170:i32)  [unwired: 11 in]
          n111 = Boolean To (0,1)(Boolean="LC_Cue_First_OnOff") -> (0, 1=w226:i16)
          n112 = Boolean To (0,1)(Boolean="LC_Cue_First_delayOpt") -> (0, 1=w225:i16)
          n113 = Boolean To (0,1)(Boolean="LC_Cue_PreR_OnOff") -> (0, 1=w224:i16)
          n114 = Boolean To (0,1)(Boolean="LC_Cue_PreR_delayOpt") -> (0, 1=w223:i16)
          n115 = Boolean To (0,1)(Boolean="LC_Cue_PostR_OnOff") -> (0, 1=w222:i16)
          n116 = Boolean To (0,1)(Boolean="LC_Cue_PostR_delayOpt") -> (0, 1=w221:i16)
          n117 = Boolean To (0,1)(Boolean="LC_Cue2_First_OnOff") -> (0, 1=w169:i16)
          n118 = Boolean To (0,1)(Boolean="LC_Cue2_First_delayOpt") -> (0, 1=w168:i16)
          n119 = Boolean To (0,1)(Boolean="LC_Cue2_PreR_OnOff") -> (0, 1=w167:i16)
          n120 = Boolean To (0,1)(Boolean="LC_Cue2_PreR_delayOpt") -> (0, 1=w166:i16)
          n121 = Boolean To (0,1)(Boolean="LC_Cue2_PostR_OnOff") -> (0, 1=w165:i16)
          n122 = Boolean To (0,1)(Boolean="LC_Cue2_PostR_delayOpt") -> (0, 1=w164:i16)
          n123 = To Unsigned Word Integer(number=w226) -> (unsigned 16bit integer=w220:u16)
          n124 = To Unsigned Word Integer(number=w225) -> (unsigned 16bit integer=w216:u16)
          n125 = To Unsigned Word Integer(number=w224) -> (unsigned 16bit integer=w214:u16)
          n126 = To Unsigned Word Integer(number=w223) -> (unsigned 16bit integer=w210:u16)
          n127 = To Unsigned Word Integer(number=w222) -> (unsigned 16bit integer=w208:u16)
          n128 = To Unsigned Word Integer(number=w221) -> (unsigned 16bit integer=w204:u16)
          n129 = To Unsigned Word Integer(number=w169) -> (unsigned 16bit integer=w157:u16)
          n130 = To Unsigned Word Integer(number=w168) -> (unsigned 16bit integer=w153:u16)
          n131 = To Unsigned Word Integer(number=w167) -> (unsigned 16bit integer=w151:u16)
          n132 = To Unsigned Word Integer(number=w166) -> (unsigned 16bit integer=w147:u16)
          n133 = To Unsigned Word Integer(number=w165) -> (unsigned 16bit integer=w145:u16)
          n134 = To Unsigned Word Integer(number=w164) -> (unsigned 16bit integer=w141:u16)
          n135 = call "BRig_dataLC_Cue_PostR_nRew1_l1.vi"() -> ("output_Cue_PostR_nRew1_l1"=w139:i32)  [unwired: 11 in]
          n136 = call "BRig_dataLC_Cue_PostR_nRew2_l1.vi"() -> ("output_Cue_PostR_nRew2_l1"=w138:i32)  [unwired: 11 in]
          n137 = call "BRig_dataLC_Cue2_PostR_nRew1_l1.vi"() -> ("output_Cue2_PostR_nRew1_l1"=w137:i32)  [unwired: 11 in]
          n138 = call "BRig_dataLC_Cue2_PostR_nRew2_l1.vi"() -> ("output_Cue2_PostR_nRew2_l1"=w136:i32)  [unwired: 11 in]
          n139 = Replace Array Subset(array=w240, new element #1=w201, index #1=w202, new element #2=w220, index #2=w238, new element #3="LC_Cue_First_Block", index #3=w237, new element #4="LC_Cue_First_Probability", index #4=w236, new element #5="LC_Cue_First_Tdelay", index #5=w235, new element #6=w216, index #6=w234, new element #7="LC_Cue_First_Count", index #7=w233, new element #8=w214, index #8=w198, new element #9="LC_Cue_PreR_Block", index #9=w197, new element #10="LC_Cue_PreR_Probability", index #10=w196, new element #11="LC_Cue_PreR_Tdelay", index #11=w195, new element #12=w210, index #12=w194, new element #13="LC_Cue_PreR_Count", index #13=w199, new element #14=w208, index #14=w200, new element #15="LC_Cue_PostR_Block", index #15=w193, new element #16="LC_Cue_PostR_Probability", index #16=w192, new element #17="LC_Cue_PostR_Tdelay", index #17=w191, new element #18=w204, index #18=w190, new element #19="LC_Cue_PostR_Count", index #19=w189, new element #20=w157, index #20=w187, new element #21="LC_Cue2_First_Block", index #21=w186, new element #22="LC_Cue2_First_Probability", index #22=w185, new element #23="LC_Cue2_First_Tdelay", index #23=w184, new element #24=w153, index #24=w183, new element #25="LC_Cue2_First_Count", index #25=w182, new element #26=w151, index #26=w181, new element #27="LC_Cue2_PreR_Block", index #27=w180, new element #28="LC_Cue2_PreR_Probability", index #28=w179, new element #29="LC_Cue2_PreR_Tdelay", index #29=w178, new element #30=w147, index #30=w177, new element #31="LC_Cue2_PreR_Count", index #31=w176, new element #32=w145, index #32=w175, new element #33="LC_Cue2_PostR_Block", index #33=w174, new element #34="LC_Cue2_PostR_Probability", index #34=w173, new element #35="LC_Cue2_PostR_Tdelay", index #35=w172, new element #36=w141, index #36=w171, new element #37="LC_Cue2_PostR_Count", index #37=w170, new element #38="LC_Cue_nRew1", index #38=w139, new element #39="LC_Cue_nRew2", index #39=w138, new element #40="LC_Cue2_nRew1", index #40=w137, new element #41="LC_Cue2_nRew2", index #41=w136) -> (w239:u16[])
        }
        frame 3 {
          n140 = call "BRig_dataLC_Selection_PostR_OnOff_l1.vi"() -> ("output_Selection_PostR_OnOff"=w257:i32)  [unwired: 11 in]
          n141 = call "BRig_dataLC_Selection_PostR_Block_l1.vi"() -> ("output_Selection_PostR_Block"=w256:i32)  [unwired: 11 in]
          n142 = call "BRig_dataLC_Selection_PostR_Prob_l1.vi"() -> ("output_Selection_PostR_Prob"=w255:i32)  [unwired: 11 in]
          n143 = call "BRig_dataLC_Selection_PostR_Delay_l1.vi"() -> ("output_Selection_PostR_Delay"=w254:i32)  [unwired: 11 in]
          n144 = call "BRig_dataLC_Selection_PostR_Count_l1.vi"() -> ("output_Selection_PostR_Count"=w253:i32)  [unwired: 11 in]
          n145 = call "BRig_dataLC_Selection_PreR_OnOff_l1.vi"() -> ("output_Selection_PreR_OnOff"=w267:i32)  [unwired: 11 in]
          n146 = call "BRig_dataLC_Selection_PreR_Block_l1.vi"() -> ("output_Selection_PreR_Block"=w266:i32)  [unwired: 11 in]
          n147 = call "BRig_dataLC_Selection_PreR_Prob_l1.vi"() -> ("output_Selection_PreR_Prob"=w265:i32)  [unwired: 11 in]
          n148 = call "BRig_dataLC_Selection_PreR_Delay_l1.vi"() -> ("output_Selection_PreR_Delay"=w264:i32)  [unwired: 11 in]
          n149 = call "BRig_dataLC_Selection_PreR_Count_l1.vi"() -> ("output_Selection_PreR_Count"=w263:i32)  [unwired: 11 in]
          n150 = call "BRig_dataLC_Selection_First_OnOff_l1.vi"() -> ("output_Selection_First_OnOff"=w277:i32)  [unwired: 11 in]
          n151 = call "BRig_dataLC_Selection_First_Block_l1.vi"() -> ("output_Selection_First_Block"=w276:i32)  [unwired: 11 in]
          n152 = call "BRig_dataLC_Selection_First_Prob_l1.vi"() -> ("output_Selection_First_Prob"=w275:i32)  [unwired: 11 in]
          n153 = call "BRig_dataLC_Selection_First_Delay_l1.vi"() -> ("output_Selection_First_Delay"=w274:i32)  [unwired: 11 in]
          n154 = call "BRig_dataLC_Selection_First_Count_l1.vi"() -> ("output_Selection_First_Count"=w273:i32)  [unwired: 11 in]
          n155 = Boolean To (0,1)(Boolean="LC_Sel_First_OnOff") -> (0, 1=w280:i16)
          n156 = Boolean To (0,1)(Boolean="LC_Sel_PreR_OnOff") -> (0, 1=w279:i16)
          n157 = Boolean To (0,1)(Boolean="LC_Sel_PostR_OnOff") -> (0, 1=w278:i16)
          n158 = To Unsigned Word Integer(number=w280) -> (unsigned 16bit integer=w272:u16)
          n159 = To Unsigned Word Integer(number=w279) -> (unsigned 16bit integer=w262:u16)
          n160 = To Unsigned Word Integer(number=w278) -> (unsigned 16bit integer=w252:u16)
          n161 = call "BRig_dataLC_Selection_PostR_nRew1_l1.vi"() -> ("output_Selection_PostR_nRew1_l1"=w244:i32)  [unwired: 11 in]
          n162 = call "BRig_dataLC_Selection_PostR_nRew2_l1.vi"() -> ("output_Selection_PostR_nRew2_l1"=w243:i32)  [unwired: 11 in]
          n163 = Replace Array Subset(array=w285, new element #1=w246, index #1=w247, new element #2=w272, index #2=w277, new element #3="LC_Sel_First_Block", index #3=w276, new element #4="LC_Sel_First_Probability", index #4=w275, new element #5="LC_Sel_First_Tdelay", index #5=w274, new element #6="LC_Sel_First_Count", index #6=w273, new element #7=w262, index #7=w267, new element #8="LC_Sel_PreR_Block", index #8=w266, new element #9="LC_Sel_PreR_Probability", index #9=w265, new element #10="LC_Sel_PreR_Tdelay", index #10=w264, new element #11="LC_Sel_PreR_Count", index #11=w263, new element #12=w252, index #12=w257, new element #13="LC_Sel_PostR_Block", index #13=w256, new element #14="LC_Sel_PostR_Probability", index #14=w255, new element #15="LC_Sel_PostR_Tdelay", index #15=w254, new element #16="LC_Sel_PostR_Count", index #16=w253, new element #17="LC_Sel_nRew1", index #17=w244, new element #18="LC_Sel_nRew2", index #18=w243) -> (w284:u16[])
        }
        frame 4 {
          n164 = call "BRig_dataLC_Reward_OnOff_l1.vi"() -> ("output_Reward_OnOff"=w320:i32)  [unwired: 11 in]
          n165 = call "BRig_dataLC_Reward_Block_l1.vi"() -> ("output_Reward_Block"=w319:i32)  [unwired: 11 in]
          n166 = call "BRig_dataLC_Reward_Trial_l1.vi"() -> ("output_Reward_Trial"=w318:i32)  [unwired: 11 in]
          n167 = call "BRig_dataLC_Reward_Prob_l1.vi"() -> ("output_Reward_Prob"=w317:i32)  [unwired: 11 in]
          n168 = call "BRig_dataLC_Reward_Delay_l1.vi"() -> ("output_Reward_Delay"=w316:i32)  [unwired: 11 in]
          n169 = call "BRig_dataLC_Wrong_OnOff_l1.vi"() -> ("output_Wrong_OnOff"=w306:i32)  [unwired: 11 in]
          n170 = call "BRig_dataLC_Wrong_Block_l1.vi"() -> ("output_Wrong_Block"=w305:i32)  [unwired: 11 in]
          n171 = call "BRig_dataLC_Wrong_Trial_l1.vi"() -> ("output_Wrong_Trial"=w304:i32)  [unwired: 11 in]
          n172 = call "BRig_dataLC_Wrong_Prob_l1.vi"() -> ("output_Wrong_Prob"=w303:i32)  [unwired: 11 in]
          n173 = call "BRig_dataLC_Wrong_Delay_l1.vi"() -> ("output_Wrong_Delay"=w302:i32)  [unwired: 11 in]
          n174 = Boolean To (0,1)(Boolean="LC_Reward_OnOff") -> (0, 1=w313:i16)
          n175 = Boolean To (0,1)(Boolean="LC_Wrong_OnOff") -> (0, 1=w312:i16)
          n176 = To Unsigned Word Integer(number=w313) -> (unsigned 16bit integer=w311:u16)
          n177 = To Unsigned Word Integer(number=w312) -> (unsigned 16bit integer=w301:u16)
          n178 = call "BRig_dataLC_Reward_nRew1_l1.vi"() -> ("output_Reward_nRew1_l1"=w293:i32)  [unwired: 11 in]
          n179 = call "BRig_dataLC_Reward_nRew2_l1.vi"() -> ("output_Reward_nRew2_l1"=w292:i32)  [unwired: 11 in]
          n180 = call "BRig_dataLC_Wrong_nRew1_l1.vi"() -> ("output_Wrong_nRew1_l1"=w289:i32)  [unwired: 11 in]
          n181 = call "BRig_dataLC_Wrong_nRew2_l1.vi"() -> ("output_Wrong_nRew2_l1"=w287:i32)  [unwired: 11 in]
          n182 = Replace Array Subset(array=w322, new element #1=w295, index #1=w296, new element #2=w311, index #2=w320, new element #3="LC_Reward_Block", index #3=w319, new element #4="LC_Reward_Trial", index #4=w318, new element #5="LC_Reward_Probability", index #5=w317, new element #6="LC_Reward_Tdelay", index #6=w316, new element #7=w301, index #7=w306, new element #8="LC_Wrong_Block", index #8=w305, new element #9="LC_Wrong_Trial", index #9=w304, new element #10="LC_Wrong_Probability", index #10=w303, new element #11="LC_Wrong_Tdelay", index #11=w302, new element #12="LC_Rew_nRew1", index #12=w293, new element #13="LC_Rew_nRew2", index #13=w292, new element #14="LC_Wro_nRew1", index #14=w289, new element #15="LC_Wro_nRew2", index #15=w287) -> (w321:u16[])
        }
        frame 5 {
          w346 = 100.0 ("y")
          n183 = call "BRig_dataExp_LED_baseline_l1.vi"() -> ("output_LED_baseline_l1"=w323:i32)  [unwired: 11 in]
          n184 = call "BRig_dataExp_L_freq_l1.vi"() -> ("output_L_freq_l1"=w345:i32)  [unwired: 11 in]
          n185 = call "BRig_dataExp_L_T_l1.vi"() -> ("output_L_T_l1"=w344:i32)  [unwired: 11 in]
          n186 = call "BRig_dataExp_L_Tpeak_l1.vi"() -> ("output_L_Tpeak_l1"=w343:i32)  [unwired: 11 in]
          n187 = call "BRig_dataExp_L_Tshutter_l1.vi"() -> ("output_L_Tshutter_l1"=w342:i32)  [unwired: 11 in]
          n188 = call "BRig_dataExp_L_power_min_l1.vi"() -> ("output_L_power_min_l1"=w341:i32)  [unwired: 11 in]
          n189 = call "BRig_dataExp_L_power_max_l1.vi"() -> ("output_L_power_max_l1"=w340:i32)  [unwired: 11 in]
          n190 = call "BRig_dataExp_L_power_step_l1.vi"() -> ("output_L_power_step_l1"=w339:i32)  [unwired: 11 in]
          n191 = call "BRig_dataExp_L_Ttotal_l1.vi"() -> ("output_L_Ttotal_l1"=w333:i32)  [unwired: 11 in]
          n192 = Boolean To (0,1)(Boolean="LED_baseline") -> (0, 1=w358:i16)
          n193 = To Unsigned Word Integer(number=w358) -> (unsigned 16bit integer=w356:u16)
          n194 = Multiply(x="Laser_power_min", y=w346) -> (x*y=w350:dbl)
          n195 = Multiply(x="Laser_power_max", y=w346) -> (x*y=w352:dbl)
          n196 = Multiply(x="Laser_power_step", y=w346) -> (x*y=w355:dbl)
          n197 = Round To Nearest(number=w350) -> (nearest integer value=w349:dbl)
          n198 = Round To Nearest(number=w352) -> (nearest integer value=w351:dbl)
          n199 = Round To Nearest(number=w355) -> (nearest integer value=w354:dbl)
          n200 = To Unsigned Word Integer(number=w349) -> (unsigned 16bit integer=w336:u16)
          n201 = To Unsigned Word Integer(number=w351) -> (unsigned 16bit integer=w337:u16)
          n202 = To Unsigned Word Integer(number=w354) -> (unsigned 16bit integer=w338:u16)
          n203 = Add(x="Laser_T", y="Laser_Tshutter") -> (x+y=w330:u16)
          n204 = Replace Array Subset(array=w327, new element=w324, index=w325) -> (w326:u16[])
          n205 = Replace Array Subset(array=w329, new element #1=w356, index #1=w323, new element #2="Laser_Freq", index #2=w345, new element #3="Laser_T", index #3=w344, new element #4="Laser_Tpeak", index #4=w343, new element #5="Laser_Tshutter", index #5=w342, new element #6=w336, index #6=w341, new element #7=w337, index #7=w340, new element #8=w338, index #8=w339, new element #9=w330, index #9=w333) -> (w328:u16[])
        }
        frame 6 {
          n206 = call "BRig_dataExp_L_freq_l1.vi"() -> ("output_L_freq_l1"=w361:i32)  [unwired: 11 in]
          n207 = call "BRig_dataExp_L_T_l1.vi"() -> ("output_L_T_l1"=w362:i32)  [unwired: 11 in]
          n208 = call "BRig_dataExp_L_Tpeak_l1.vi"() -> ("output_L_Tpeak_l1"=w360:i32)  [unwired: 11 in]
          n209 = call "BRig_dataExp_L_Tshutter_l1.vi"() -> ("output_L_Tshutter_l1"=w359:i32)  [unwired: 11 in]
          n210 = Replace Array Subset(array=w366, new element=w363, index=w364) -> (w365:u16[])
          n211 = call "BRig_RT__Case_Idle__calc_LaserPulse.vi"("input_dataExp_L_Tshutter"=w359, "input_dataExp_L_Tpeak"=w360, "input_dataExp_L_T"=w362, "input_dataExp_L_freq"=w361, "input_dataExp"=w368) -> ("output_cluster"=→"LaserPulseTrain":cluster{u16[], u16[]})  [unwired: 6 in]
        }
      }
    }
    frame True {
      w497 = 100.0 ("y")
      n212 = call "BRig_dataLC_ENL_First_OnOff_l1.vi"() -> ("output_ENL_First_OnOff"=w639:i32)  [unwired: 11 in]
      n213 = call "BRig_dataLC_ENL_First_Block_l1.vi"() -> ("output_ENL_First_Block"=w638:i32)  [unwired: 11 in]
      n214 = call "BRig_dataLC_ENL_First_Prob_l1.vi"() -> ("output_ENL_First_Prob"=w637:i32)  [unwired: 11 in]
      n215 = call "BRig_dataLC_ENL_First_Delay_l1.vi"() -> ("output_ENL_First_Delay"=w636:i32)  [unwired: 11 in]
      n216 = call "BRig_dataLC_ENL_First_DelayOpt_l1.vi"() -> ("output_ENL_First_DelayOpt"=w635:i32)  [unwired: 11 in]
      n217 = call "BRig_dataLC_ENL_First_Count_l1.vi"() -> ("output_ENL_First_Count"=w634:i32)  [unwired: 11 in]
      n218 = call "BRig_dataLC_ENL_PreR_OnOff_l1.vi"() -> ("output_ENL_PreR_OnOff"=w633:i32)  [unwired: 11 in]
      n219 = call "BRig_dataLC_ENL_PreR_Block_l1.vi"() -> ("output_ENL_PreR_Block"=w632:i32)  [unwired: 11 in]
      n220 = call "BRig_dataLC_ENL_PreR_Prob_l1.vi"() -> ("output_ENL_PreR_Prob"=w631:i32)  [unwired: 11 in]
      n221 = call "BRig_dataLC_ENL_PreR_Delay_l1.vi"() -> ("output_ENL_PreR_Delay"=w630:i32)  [unwired: 11 in]
      n222 = call "BRig_dataLC_ENL_PreR_DelayOpt_l1.vi"() -> ("output_ENL_PreR_DelayOpt"=w629:i32)  [unwired: 11 in]
      n223 = call "BRig_dataLC_ENL_PreR_Count_l1.vi"() -> ("output_ENL_PreR_Count"=w628:i32)  [unwired: 11 in]
      n224 = call "BRig_dataLC_ENL_PostR_OnOff_l1.vi"() -> ("output_ENL_PostR_OnOff"=w627:i32)  [unwired: 11 in]
      n225 = call "BRig_dataLC_ENL_PostR_Block_l1.vi"() -> ("output_ENL_PostR_Block"=w626:i32)  [unwired: 11 in]
      n226 = call "BRig_dataLC_ENL_PostR_Prob_l1.vi"() -> ("output_ENL_PostR_Prob"=w625:i32)  [unwired: 11 in]
      n227 = call "BRig_dataLC_ENL_PostR_Delay_l1.vi"() -> ("output_ENL_PostR_Delay"=w624:i32)  [unwired: 11 in]
      n228 = call "BRig_dataLC_ENL_PostR_DelayOpt_l1.vi"() -> ("output_ENL_PostR_DelayOpt"=w623:i32)  [unwired: 11 in]
      n229 = call "BRig_dataLC_ENL_PostR_Count_l1.vi"() -> ("output_ENL_PostR_Count"=w622:i32)  [unwired: 11 in]
      n230 = call "BRig_dataLC_Reward_nRew1_l1.vi"() -> ("output_Reward_nRew1_l1"=w376:i32)  [unwired: 11 in]
      n231 = call "BRig_dataLC_Reward_nRew2_l1.vi"() -> ("output_Reward_nRew2_l1"=w375:i32)  [unwired: 11 in]
      n232 = call "BRig_dataLC_Wrong_nRew1_l1.vi"() -> ("output_Wrong_nRew1_l1"=w372:i32)  [unwired: 11 in]
      n233 = call "BRig_dataLC_Wrong_nRew2_l1.vi"() -> ("output_Wrong_nRew2_l1"=w371:i32)  [unwired: 11 in]
      n234 = call "BRig_dataLC_ENL2_First_OnOff_l1.vi"() -> ("output_ENL2_First_OnOff"=w482:i32)  [unwired: 11 in]
      n235 = call "BRig_dataLC_ENL2_First_Block_l1.vi"() -> ("output_ENL2_First_Block"=w481:i32)  [unwired: 11 in]
      n236 = call "BRig_dataLC_ENL2_First_Prob_l1.vi"() -> ("output_ENL2_First_Prob"=w480:i32)  [unwired: 11 in]
      n237 = call "BRig_dataLC_ENL2_First_Delay_l1.vi"() -> ("output_ENL2_First_Delay"=w479:i32)  [unwired: 11 in]
      n238 = call "BRig_dataLC_ENL2_First_DelayOpt_l1.vi"() -> ("output_ENL2_First_DelayOpt"=w478:i32)  [unwired: 11 in]
      n239 = call "BRig_dataLC_ENL2_First_Count_l1.vi"() -> ("output_ENL2_First_Count"=w477:i32)  [unwired: 11 in]
      n240 = call "BRig_dataLC_ENL2_PreR_OnOff_l1.vi"() -> ("output_ENL2_PreR_OnOff"=w476:i32)  [unwired: 11 in]
      n241 = call "BRig_dataLC_ENL2_PreR_Block_l1.vi"() -> ("output_ENL2_PreR_Block"=w475:i32)  [unwired: 11 in]
      n242 = call "BRig_dataLC_ENL2_PreR_Prob_l1.vi"() -> ("output_ENL2_PreR_Prob"=w474:i32)  [unwired: 11 in]
      n243 = call "BRig_dataLC_ENL2_PreR_Delay_l1.vi"() -> ("output_ENL2_PreR_Delay"=w473:i32)  [unwired: 11 in]
      n244 = call "BRig_dataLC_ENL2_PreR_DelayOpt_l1.vi"() -> ("output_ENL2_PreR_DelayOpt"=w472:i32)  [unwired: 11 in]
      n245 = call "BRig_dataLC_ENL2_PreR_Count_l1.vi"() -> ("output_ENL2_PreR_Count"=w471:i32)  [unwired: 11 in]
      n246 = call "BRig_dataLC_ENL2_PostR_OnOff_l1.vi"() -> ("output_ENL2_PostR_OnOff"=w470:i32)  [unwired: 11 in]
      n247 = call "BRig_dataLC_ENL2_PostR_Block_l1.vi"() -> ("output_ENL2_PostR_Block"=w469:i32)  [unwired: 11 in]
      n248 = call "BRig_dataLC_ENL2_PostR_Prob_l1.vi"() -> ("output_ENL2_PostR_Prob"=w468:i32)  [unwired: 11 in]
      n249 = call "BRig_dataLC_ENL2_PostR_Delay_l1.vi"() -> ("output_ENL2_PostR_Delay"=w467:i32)  [unwired: 11 in]
      n250 = call "BRig_dataLC_ENL2_PostR_DelayOpt_l1.vi"() -> ("output_ENL2_PostR_DelayOpt"=w466:i32)  [unwired: 11 in]
      n251 = call "BRig_dataLC_ENL2_PostR_Count_l1.vi"() -> ("output_ENL2_PostR_Count"=w465:i32)  [unwired: 11 in]
      n252 = Index Array(array=w377, index #1=w376, index #2=w375, index #3=w372, index #4=w371) -> (element #1=w374:u16, element #2=w373:u16, element #3=w370:u16, element #4=w369:u16)
      n253 = Index Array(array=w377, index #1=w639, index #2=w638, index #3=w637, index #4=w636, index #5=w635, index #6=w634, index #7=w633, index #8=w632, index #9=w631, index #10=w630, index #11=w629, index #12=w628, index #13=w627, index #14=w626, index #15=w625, index #16=w624, index #17=w623, index #18=w622) -> (element #1=w615:u16, element #2=w614:u16, element #3=w613:u16, element #4=w612:u16, element #5=w611:u16, element #6=w610:u16, element #7=w609:u16, element #8=w608:u16, element #9=w607:u16, element #10=w606:u16, element #11=w605:u16, element #12=w604:u16, element #13=w603:u16, element #14=w602:u16, element #15=w601:u16, element #16=w600:u16, element #17=w599:u16, element #18=w598:u16)
      n254 = local write "LC_Rew_nRew1"(w374) -> ()
      n255 = local write "LC_Rew_nRew2"(w373) -> ()
      n256 = local write "LC_Wro_nRew1"(w370) -> ()
      n257 = local write "LC_Wro_nRew2"(w369) -> ()
      n258 = Index Array(array=w377, index #1=w482, index #2=w481, index #3=w480, index #4=w479, index #5=w478, index #6=w477, index #7=w476, index #8=w475, index #9=w474, index #10=w473, index #11=w472, index #12=w471, index #13=w470, index #14=w469, index #15=w468, index #16=w467, index #17=w466, index #18=w465) -> (element #1=w441:u16, element #2=w442:u16, element #3=w443:u16, element #4=w444:u16, element #5=w445:u16, element #6=w446:u16, element #7=w447:u16, element #8=w448:u16, element #9=w449:u16, element #10=w450:u16, element #11=w451:u16, element #12=w452:u16, element #13=w454:u16, element #14=w455:u16, element #15=w456:u16, element #16=w457:u16, element #17=w458:u16, element #18=w459:u16)
      n259 = Not Equal To 0?(x=w615) -> (x != 0?=w621:bool)
      n260 = Not Equal To 0?(x=w611) -> (x != 0?=w620:bool)
      n261 = Not Equal To 0?(x=w609) -> (x != 0?=w619:bool)
      n262 = Not Equal To 0?(x=w605) -> (x != 0?=w618:bool)
      n263 = Not Equal To 0?(x=w603) -> (x != 0?=w617:bool)
      n264 = Not Equal To 0?(x=w599) -> (x != 0?=w616:bool)
      n265 = local write "LC_ENL_First_OnOff"(w621) -> ()
      n266 = local write "LC_ENL_First_Block"(w614) -> ()
      n267 = local write "LC_ENL_First_Probability"(w613) -> ()
      n268 = local write "LC_ENL_First_Tdelay"(w612) -> ()
      n269 = local write "LC_ENL_First_delayOpt"(w620) -> ()
      n270 = local write "LC_ENL_First_Count"(w610) -> ()
      n271 = local write "LC_ENL_PreR_OnOff"(w619) -> ()
      n272 = local write "LC_ENL_PreR_Block"(w608) -> ()
      n273 = local write "LC_ENL_PreR_Probability"(w607) -> ()
      n274 = local write "LC_ENL_PreR_Tdelay"(w606) -> ()
      n275 = local write "LC_ENL_PreR_delayOpt"(w618) -> ()
      n276 = local write "LC_ENL_PreR_Count"(w604) -> ()
      n277 = local write "LC_ENL_PostR_OnOff"(w617) -> ()
      n278 = local write "LC_ENL_PostR_Block"(w602) -> ()
      n279 = local write "LC_ENL_PostR_Probability"(w601) -> ()
      n280 = local write "LC_ENL_PostR_Tdelay"(w600) -> ()
      n281 = local write "LC_ENL_PostR_delayOpt"(w616) -> ()
      n282 = local write "LC_ENL_PostR_Count"(w598) -> ()
      n283 = Not Equal To 0?(x=w441) -> (x != 0?=w462:bool)
      n284 = Not Equal To 0?(x=w445) -> (x != 0?=w463:bool)
      n285 = Not Equal To 0?(x=w447) -> (x != 0?=w461:bool)
      n286 = Not Equal To 0?(x=w451) -> (x != 0?=w464:bool)
      n287 = Not Equal To 0?(x=w454) -> (x != 0?=w460:bool)
      n288 = Not Equal To 0?(x=w458) -> (x != 0?=w453:bool)
      n289 = local write "LC_ENL2_First_OnOff"(w462) -> ()
      n290 = local write "LC_ENL2_First_Block"(w442) -> ()
      n291 = local write "LC_ENL2_First_Probability"(w443) -> ()
      n292 = local write "LC_ENL2_First_Tdelay"(w444) -> ()
      n293 = local write "LC_ENL2_First_delayOpt"(w463) -> ()
      n294 = local write "LC_ENL2_First_Count"(w446) -> ()
      n295 = local write "LC_ENL2_PreR_OnOff"(w461) -> ()
      n296 = local write "LC_ENL2_PreR_Block"(w448) -> ()
      n297 = local write "LC_ENL2_PreR_Probability"(w449) -> ()
      n298 = local write "LC_ENL2_PreR_Tdelay"(w450) -> ()
      n299 = local write "LC_ENL2_PreR_delayOpt"(w464) -> ()
      n300 = local write "LC_ENL2_PreR_Count"(w452) -> ()
      n301 = local write "LC_ENL2_PostR_OnOff"(w460) -> ()
      n302 = local write "LC_ENL2_PostR_Block"(w455) -> ()
      n303 = local write "LC_ENL2_PostR_Probability"(w456) -> ()
      n304 = local write "LC_ENL2_PostR_Tdelay"(w457) -> ()
      n305 = local write "LC_ENL2_PostR_delayOpt"(w453) -> ()
      n306 = local write "LC_ENL2_PostR_Count"(w459) -> ()
      n307 = call "BRig_dataLC_Cue_PreR_OnOff_l1.vi"() -> ("output_Cue_PreR_OnOff"=w487:i32)  [unwired: 11 in]
      n308 = call "BRig_dataLC_Cue_PreR_Block_l1.vi"() -> ("output_Cue_PreR_Block"=w486:i32)  [unwired: 11 in]
      n309 = call "BRig_dataLC_Cue_PreR_Prob_l1.vi"() -> ("output_Cue_PreR_Prob"=w485:i32)  [unwired: 11 in]
      n310 = call "BRig_dataLC_Cue_PreR_Delay_l1.vi"() -> ("output_Cue_PreR_Delay"=w484:i32)  [unwired: 11 in]
      n311 = call "BRig_dataLC_Cue_PreR_DelayOpt_l1.vi"() -> ("output_Cue_PreR_DelayOpt"=w483:i32)  [unwired: 11 in]
      n312 = call "BRig_dataLC_Cue_PreR_Count_l1.vi"() -> ("output_Cue_PreR_Count"=w488:i32)  [unwired: 11 in]
      n313 = call "BRig_dataLC_Cue_First_OnOff_l1.vi"() -> ("output_Cue_First_OnOff"=w645:i32)  [unwired: 11 in]
      n314 = call "BRig_dataLC_Cue_First_Block_l1.vi"() -> ("output_Cue_First_Block"=w644:i32)  [unwired: 11 in]
      n315 = call "BRig_dataLC_Cue_First_Prob_l1.vi"() -> ("output_Cue_First_Prob"=w643:i32)  [unwired: 11 in]
      n316 = call "BRig_dataLC_Cue_First_Delay_l1.vi"() -> ("output_Cue_First_Delay"=w642:i32)  [unwired: 11 in]
      n317 = call "BRig_dataLC_Cue_First_DelayOpt_l1.vi"() -> ("output_Cue_First_DelayOpt"=w641:i32)  [unwired: 11 in]
      n318 = call "BRig_dataLC_Cue_First_Count_l1.vi"() -> ("output_Cue_First_Count"=w640:i32)  [unwired: 11 in]
      n319 = call "BRig_dataLC_Cue_PostR_OnOff_l1.vi"() -> ("output_Cue_PostR_OnOff"=w493:i32)  [unwired: 11 in]
      n320 = call "BRig_dataLC_Cue_PostR_Block_l1.vi"() -> ("output_Cue_PostR_Block"=w492:i32)  [unwired: 11 in]
      n321 = call "BRig_dataLC_Cue_PostR_Prob_l1.vi"() -> ("output_Cue_PostR_Prob"=w491:i32)  [unwired: 11 in]
      n322 = call "BRig_dataLC_Cue_PostR_Delay_l1.vi"() -> ("output_Cue_PostR_Delay"=w490:i32)  [unwired: 11 in]
      n323 = call "BRig_dataLC_Cue_PostR_DelayOpt_l1.vi"() -> ("output_Cue_PostR_DelayOpt"=w489:i32)  [unwired: 11 in]
      n324 = call "BRig_dataLC_Cue_PostR_Count_l1.vi"() -> ("output_Cue_PostR_Count"=w494:i32)  [unwired: 11 in]
      n325 = call "BRig_dataExp_LED_baseline_Cue.vi"() -> ("output_LED_baseline_Cue"=w518:i32)  [unwired: 11 in]
      n326 = call "BRig_dataExp_L_freq_l1.vi"() -> ("output_L_freq_l1"=w517:i32)  [unwired: 11 in]
      n327 = call "BRig_dataExp_L_T_l1.vi"() -> ("output_L_T_l1"=w516:i32)  [unwired: 11 in]
      n328 = call "BRig_dataExp_L_Tpeak_l1.vi"() -> ("output_L_Tpeak_l1"=w515:i32)  [unwired: 11 in]
      n329 = call "BRig_dataExp_L_Tshutter_l1.vi"() -> ("output_L_Tshutter_l1"=w514:i32)  [unwired: 11 in]
      n330 = call "BRig_dataExp_L_power_min_l1.vi"() -> ("output_L_power_min_l1"=w513:i32)  [unwired: 11 in]
      n331 = call "BRig_dataExp_L_power_max_l1.vi"() -> ("output_L_power_max_l1"=w512:i32)  [unwired: 11 in]
      n332 = call "BRig_dataExp_L_power_step_l1.vi"() -> ("output_L_power_step_l1"=w511:i32)  [unwired: 11 in]
      n333 = Index Array(array=w377, index #1=w645, index #2=w644, index #3=w643, index #4=w642, index #5=w641, index #6=w640, index #7=w487, index #8=w486, index #9=w485, index #10=w484, index #11=w483, index #12=w488, index #13=w493, index #14=w492, index #15=w491, index #16=w490, index #17=w489, index #18=w494) -> (element #1=w591:u16, element #2=w590:u16, element #3=w589:u16, element #4=w588:u16, element #5=w587:u16, element #6=w586:u16, element #7=w585:u16, element #8=w584:u16, element #9=w583:u16, element #10=w582:u16, element #11=w581:u16, element #12=w580:u16, element #13=w579:u16, element #14=w578:u16, element #15=w577:u16, element #16=w576:u16, element #17=w575:u16, element #18=w574:u16)
      n334 = Index Array(array=w394, index #1=w518, index #2=w517, index #3=w516, index #4=w515, index #5=w514, index #6=w513, index #7=w512, index #8=w511) -> (element #1=w510:u16, element #2=w508:u16, element #3=w507:u16, element #4=w506:u16, element #5=w505:u16, element #6=w504:u16, element #7=w503:u16, element #8=w502:u16)
      n335 = To Double Precision Float(number=w504) -> (double precision float=w501:dbl)
      n336 = To Double Precision Float(number=w503) -> (double precision float=w496:dbl)
      n337 = To Double Precision Float(number=w502) -> (double precision float=w495:dbl)
      n338 = Not Equal To 0?(x=w591) -> (x != 0?=w597:bool)
      n339 = Not Equal To 0?(x=w587) -> (x != 0?=w596:bool)
      n340 = Not Equal To 0?(x=w585) -> (x != 0?=w595:bool)
      n341 = Not Equal To 0?(x=w581) -> (x != 0?=w594:bool)
      n342 = Not Equal To 0?(x=w579) -> (x != 0?=w593:bool)
      n343 = Not Equal To 0?(x=w575) -> (x != 0?=w592:bool)
      n344 = Divide(x=w501, y=w497) -> (x/y=w500:dbl)
      n345 = Divide(x=w496, y=w497) -> (x/y=w499:dbl)
      n346 = Divide(x=w495, y=w497) -> (x/y=w498:dbl)
      n347 = local write "LC_Cue_First_OnOff"(w597) -> ()
      n348 = local write "LC_Cue_First_Block"(w590) -> ()
      n349 = local write "LC_Cue_First_Probability"(w589) -> ()
      n350 = local write "LC_Cue_First_Tdelay"(w588) -> ()
      n351 = local write "LC_Cue_First_delayOpt"(w596) -> ()
      n352 = local write "LC_Cue_First_Count"(w586) -> ()
      n353 = local write "LC_Cue_PreR_OnOff"(w595) -> ()
      n354 = local write "LC_Cue_PreR_Block"(w584) -> ()
      n355 = local write "LC_Cue_PreR_Probability"(w583) -> ()
      n356 = local write "LC_Cue_PreR_Tdelay"(w582) -> ()
      n357 = local write "LC_Cue_PreR_delayOpt"(w594) -> ()
      n358 = local write "LC_Cue_PreR_Count"(w580) -> ()
      n359 = local write "LC_Cue_PostR_OnOff"(w593) -> ()
      n360 = local write "LC_Cue_PostR_Block"(w578) -> ()
      n361 = local write "LC_Cue_PostR_Probability"(w577) -> ()
      n362 = local write "LC_Cue_PostR_Tdelay"(w576) -> ()
      n363 = local write "LC_Cue_PostR_delayOpt"(w592) -> ()
      n364 = local write "LC_Cue_PostR_Count"(w574) -> ()
      n365 = Not Equal To 0?(x=w510) -> (x != 0?=w509:bool)
      n366 = call "BRig_dataLC_Cue2_First_OnOff_l1.vi"() -> ("output_Cue2_First_OnOff"=w417:i32)  [unwired: 11 in]
      n367 = call "BRig_dataLC_Cue2_First_Block_l1.vi"() -> ("output_Cue2_First_Block"=w418:i32)  [unwired: 11 in]
      n368 = call "BRig_dataLC_Cue2_First_Prob_l1.vi"() -> ("output_Cue2_First_Prob"=w419:i32)  [unwired: 11 in]
      n369 = call "BRig_dataLC_Cue2_First_Delay_l1.vi"() -> ("output_Cue2_First_Delay"=w420:i32)  [unwired: 11 in]
      n370 = call "BRig_dataLC_Cue2_First_DelayOpt_l1.vi"() -> ("output_Cue2_First_DelayOpt"=w421:i32)  [unwired: 11 in]
      n371 = call "BRig_dataLC_Cue2_First_Count_l1.vi"() -> ("output_Cue2_First_Count"=w422:i32)  [unwired: 11 in]
      n372 = call "BRig_dataLC_Cue2_PreR_OnOff_l1.vi"() -> ("output_Cue2_PreR_OnOff"=w423:i32)  [unwired: 11 in]
      n373 = call "BRig_dataLC_Cue2_PreR_Block_l1.vi"() -> ("output_Cue2_PreR_Block"=w424:i32)  [unwired: 11 in]
      n374 = call "BRig_dataLC_Cue2_PreR_Prob_l1.vi"() -> ("output_Cue2_PreR_Prob"=w425:i32)  [unwired: 11 in]
      n375 = call "BRig_dataLC_Cue2_PreR_Delay_l1.vi"() -> ("output_Cue2_PreR_Delay"=w426:i32)  [unwired: 11 in]
      n376 = call "BRig_dataLC_Cue2_PreR_DelayOpt_l1.vi"() -> ("output_Cue2_PreR_DelayOpt"=w427:i32)  [unwired: 11 in]
      n377 = call "BRig_dataLC_Cue2_PreR_Count_l1.vi"() -> ("output_Cue2_PreR_Count"=w428:i32)  [unwired: 11 in]
      n378 = call "BRig_dataLC_Cue2_PostR_OnOff_l1.vi"() -> ("output_Cue2_PostR_OnOff"=w429:i32)  [unwired: 11 in]
      n379 = call "BRig_dataLC_Cue2_PostR_Block_l1.vi"() -> ("output_Cue2_PostR_Block"=w430:i32)  [unwired: 11 in]
      n380 = call "BRig_dataLC_Cue2_PostR_Prob_l1.vi"() -> ("output_Cue2_PostR_Prob"=w431:i32)  [unwired: 11 in]
      n381 = call "BRig_dataLC_Cue2_PostR_Delay_l1.vi"() -> ("output_Cue2_PostR_Delay"=w432:i32)  [unwired: 11 in]
      n382 = call "BRig_dataLC_Cue2_PostR_DelayOpt_l1.vi"() -> ("output_Cue2_PostR_DelayOpt"=w433:i32)  [unwired: 11 in]
      n383 = call "BRig_dataLC_Cue2_PostR_Count_l1.vi"() -> ("output_Cue2_PostR_Count"=w434:i32)  [unwired: 11 in]
      n384 = local write "LED_baseline"(w509) -> ()
      n385 = local write "Laser_Freq"(w508) -> ()
      n386 = local write "Laser_T"(w507) -> ()
      n387 = local write "Laser_Tpeak"(w506) -> ()
      n388 = local write "Laser_Tshutter"(w505) -> ()
      n389 = local write "Laser_power_min"(w500) -> ()
      n390 = local write "Laser_power_max"(w499) -> ()
      n391 = local write "Laser_power_step"(w498) -> ()
      n392 = Index Array(array=w377, index #1=w417, index #2=w418, index #3=w419, index #4=w420, index #5=w421, index #6=w422, index #7=w423, index #8=w424, index #9=w425, index #10=w426, index #11=w427, index #12=w428, index #13=w429, index #14=w430, index #15=w431, index #16=w432, index #17=w433, index #18=w434) -> (element #1=w435:u16, element #2=w413:u16, element #3=w412:u16, element #4=w411:u16, element #5=w436:u16, element #6=w414:u16, element #7=w437:u16, element #8=w408:u16, element #9=w407:u16, element #10=w406:u16, element #11=w438:u16, element #12=w405:u16, element #13=w439:u16, element #14=w402:u16, element #15=w401:u16, element #16=w400:u16, element #17=w440:u16, element #18=w399:u16)
      n393 = call "BRig_dataLC_Selection_PostR_OnOff_l1.vi"() -> ("output_Selection_PostR_OnOff"=w563:i32)  [unwired: 11 in]
      n394 = call "BRig_dataLC_Selection_PostR_Block_l1.vi"() -> ("output_Selection_PostR_Block"=w562:i32)  [unwired: 11 in]
      n395 = call "BRig_dataLC_Selection_PostR_Prob_l1.vi"() -> ("output_Selection_PostR_Prob"=w561:i32)  [unwired: 11 in]
      n396 = call "BRig_dataLC_Selection_PostR_Delay_l1.vi"() -> ("output_Selection_PostR_Delay"=w560:i32)  [unwired: 11 in]
      n397 = call "BRig_dataLC_Selection_PostR_Count_l1.vi"() -> ("output_Selection_PostR_Count"=w559:i32)  [unwired: 11 in]
      n398 = call "BRig_dataLC_Selection_PreR_OnOff_l1.vi"() -> ("output_Selection_PreR_OnOff"=w568:i32)  [unwired: 11 in]
      n399 = call "BRig_dataLC_Selection_PreR_Block_l1.vi"() -> ("output_Selection_PreR_Block"=w567:i32)  [unwired: 11 in]
      n400 = call "BRig_dataLC_Selection_PreR_Prob_l1.vi"() -> ("output_Selection_PreR_Prob"=w566:i32)  [unwired: 11 in]
      n401 = call "BRig_dataLC_Selection_PreR_Delay_l1.vi"() -> ("output_Selection_PreR_Delay"=w565:i32)  [unwired: 11 in]
      n402 = call "BRig_dataLC_Selection_PreR_Count_l1.vi"() -> ("output_Selection_PreR_Count"=w564:i32)  [unwired: 11 in]
      n403 = call "BRig_dataLC_Selection_First_OnOff_l1.vi"() -> ("output_Selection_First_OnOff"=w573:i32)  [unwired: 11 in]
      n404 = call "BRig_dataLC_Selection_First_Block_l1.vi"() -> ("output_Selection_First_Block"=w572:i32)  [unwired: 11 in]
      n405 = call "BRig_dataLC_Selection_First_Prob_l1.vi"() -> ("output_Selection_First_Prob"=w571:i32)  [unwired: 11 in]
      n406 = call "BRig_dataLC_Selection_First_Delay_l1.vi"() -> ("output_Selection_First_Delay"=w570:i32)  [unwired: 11 in]
      n407 = call "BRig_dataLC_Selection_First_Count_l1.vi"() -> ("output_Selection_First_Count"=w569:i32)  [unwired: 11 in]
      n408 = call "BRig_dataLC_Reward_OnOff_l1.vi"() -> ("output_Reward_OnOff"=w540:i32)  [unwired: 11 in]
      n409 = call "BRig_dataLC_Reward_Block_l1.vi"() -> ("output_Reward_Block"=w539:i32)  [unwired: 11 in]
      n410 = call "BRig_dataLC_Reward_Trial_l1.vi"() -> ("output_Reward_Trial"=w538:i32)  [unwired: 11 in]
      n411 = call "BRig_dataLC_Reward_Prob_l1.vi"() -> ("output_Reward_Prob"=w537:i32)  [unwired: 11 in]
      n412 = call "BRig_dataLC_Reward_Delay_l1.vi"() -> ("output_Reward_Delay"=w536:i32)  [unwired: 11 in]
      n413 = call "BRig_dataLC_Wrong_OnOff_l1.vi"() -> ("output_Wrong_OnOff"=w535:i32)  [unwired: 11 in]
      n414 = call "BRig_dataLC_Wrong_Block_l1.vi"() -> ("output_Wrong_Block"=w534:i32)  [unwired: 11 in]
      n415 = call "BRig_dataLC_Wrong_Trial_l1.vi"() -> ("output_Wrong_Trial"=w533:i32)  [unwired: 11 in]
      n416 = call "BRig_dataLC_Wrong_Prob_l1.vi"() -> ("output_Wrong_Prob"=w532:i32)  [unwired: 11 in]
      n417 = call "BRig_dataLC_Wrong_Delay_l1.vi"() -> ("output_Wrong_Delay"=w531:i32)  [unwired: 11 in]
      n418 = Not Equal To 0?(x=w435) -> (x != 0?=w416:bool)
      n419 = Not Equal To 0?(x=w436) -> (x != 0?=w415:bool)
      n420 = Not Equal To 0?(x=w437) -> (x != 0?=w409:bool)
      n421 = Not Equal To 0?(x=w438) -> (x != 0?=w410:bool)
      n422 = Not Equal To 0?(x=w439) -> (x != 0?=w404:bool)
      n423 = Not Equal To 0?(x=w440) -> (x != 0?=w403:bool)
      n424 = call "BRig_dataLC_ENL_PostR_nRew1_l1.vi"() -> ("output_ENL_PostR_nRew1_l1"=w398:i32)  [unwired: 11 in]
      n425 = call "BRig_dataLC_ENL_PostR_nRew2_l1.vi"() -> ("output_ENL_PostR_nRew2_l1"=w397:i32)  [unwired: 11 in]
      n426 = call "BRig_dataLC_ENL2_PostR_nRew1_l1.vi"() -> ("output_ENL2_PostR_nRew1_l1"=w393:i32)  [unwired: 11 in]
      n427 = call "BRig_dataLC_ENL2_PostR_nRew2_l1.vi"() -> ("output_ENL2_PostR_nRew2_l1"=w392:i32)  [unwired: 11 in]
      n428 = call "BRig_dataLC_Cue_PostR_nRew1_l1.vi"() -> ("output_Cue_PostR_nRew1_l1"=w389:i32)  [unwired: 11 in]
      n429 = call "BRig_dataLC_Cue_PostR_nRew2_l1.vi"() -> ("output_Cue_PostR_nRew2_l1"=w388:i32)  [unwired: 11 in]
      n430 = call "BRig_dataLC_Cue2_PostR_nRew1_l1.vi"() -> ("output_Cue2_PostR_nRew1_l1"=w387:i32)  [unwired: 11 in]
      n431 = call "BRig_dataLC_Cue2_PostR_nRew2_l1.vi"() -> ("output_Cue2_PostR_nRew2_l1"=w386:i32)  [unwired: 11 in]
      n432 = call "BRig_dataLC_Selection_PostR_nRew1_l1.vi"() -> ("output_Selection_PostR_nRew1_l1"=w385:i32)  [unwired: 11 in]
      n433 = call "BRig_dataLC_Selection_PostR_nRew2_l1.vi"() -> ("output_Selection_PostR_nRew2_l1"=w384:i32)  [unwired: 11 in]
      n434 = Index Array(array=w377, index #1=w540, index #2=w539, index #3=w538, index #4=w537, index #5=w536, index #6=w535, index #7=w534, index #8=w533, index #9=w532, index #10=w531) -> (element #1=w528:u16, element #2=w527:u16, element #3=w526:u16, element #4=w525:u16, element #5=w524:u16, element #6=w523:u16, element #7=w522:u16, element #8=w521:u16, element #9=w520:u16, element #10=w519:u16)
      n435 = local write "LC_Cue2_First_OnOff"(w416) -> ()
      n436 = local write "LC_Cue2_First_Block"(w413) -> ()
      n437 = local write "LC_Cue2_First_Probability"(w412) -> ()
      n438 = local write "LC_Cue2_First_Tdelay"(w411) -> ()
      n439 = local write "LC_Cue2_First_delayOpt"(w415) -> ()
      n440 = local write "LC_Cue2_First_Count"(w414) -> ()
      n441 = local write "LC_Cue2_PreR_OnOff"(w409) -> ()
      n442 = local write "LC_Cue2_PreR_Block"(w408) -> ()
      n443 = local write "LC_Cue2_PreR_Probability"(w407) -> ()
      n444 = local write "LC_Cue2_PreR_Tdelay"(w406) -> ()
      n445 = local write "LC_Cue2_PreR_delayOpt"(w410) -> ()
      n446 = local write "LC_Cue2_PreR_Count"(w405) -> ()
      n447 = local write "LC_Cue2_PostR_OnOff"(w404) -> ()
      n448 = local write "LC_Cue2_PostR_Block"(w402) -> ()
      n449 = local write "LC_Cue2_PostR_Probability"(w401) -> ()
      n450 = local write "LC_Cue2_PostR_Tdelay"(w400) -> ()
      n451 = local write "LC_Cue2_PostR_delayOpt"(w403) -> ()
      n452 = local write "LC_Cue2_PostR_Count"(w399) -> ()
      n453 = Index Array(array=w377, index #1=w573, index #2=w572, index #3=w571, index #4=w570, index #5=w569, index #6=w568, index #7=w567, index #8=w566, index #9=w565, index #10=w564, index #11=w563, index #12=w562, index #13=w561, index #14=w560, index #15=w559) -> (element #1=w555:u16, element #2=w554:u16, element #3=w553:u16, element #4=w552:u16, element #5=w551:u16, element #6=w550:u16, element #7=w549:u16, element #8=w548:u16, element #9=w547:u16, element #10=w546:u16, element #11=w545:u16, element #12=w544:u16, element #13=w543:u16, element #14=w542:u16, element #15=w541:u16)
      n454 = Not Equal To 0?(x=w528) -> (x != 0?=w530:bool)
      n455 = Not Equal To 0?(x=w523) -> (x != 0?=w529:bool)
      n456 = Not Equal To 0?(x=w555) -> (x != 0?=w558:bool)
      n457 = Not Equal To 0?(x=w550) -> (x != 0?=w557:bool)
      n458 = Not Equal To 0?(x=w545) -> (x != 0?=w556:bool)
      n459 = Index Array(array=w377, index #1=w398, index #2=w397, index #3=w393, index #4=w392, index #5=w389, index #6=w388, index #7=w387, index #8=w386, index #9=w385, index #10=w384) -> (element #1=w396:u16, element #2=w395:u16, element #3=w391:u16, element #4=w390:u16, element #5=w383:u16, element #6=w382:u16, element #7=w381:u16, element #8=w380:u16, element #9=w379:u16, element #10=w378:u16)
      n460 = local write "LC_Reward_OnOff"(w530) -> ()
      n461 = local write "LC_Reward_Block"(w527) -> ()
      n462 = local write "LC_Reward_Trial"(w526) -> ()
      n463 = local write "LC_Reward_Probability"(w525) -> ()
      n464 = local write "LC_Reward_Tdelay"(w524) -> ()
      n465 = local write "LC_Wrong_OnOff"(w529) -> ()
      n466 = local write "LC_Wrong_Block"(w522) -> ()
      n467 = local write "LC_Wrong_Trial"(w521) -> ()
      n468 = local write "LC_Wrong_Probability"(w520) -> ()
      n469 = local write "LC_Wrong_Tdelay"(w519) -> ()
      n470 = local write "LC_Sel_First_OnOff"(w558) -> ()
      n471 = local write "LC_Sel_First_Block"(w554) -> ()
      n472 = local write "LC_Sel_First_Probability"(w553) -> ()
      n473 = local write "LC_Sel_First_Tdelay"(w552) -> ()
      n474 = local write "LC_Sel_First_Count"(w551) -> ()
      n475 = local write "LC_Sel_PreR_OnOff"(w557) -> ()
      n476 = local write "LC_Sel_PreR_Block"(w549) -> ()
      n477 = local write "LC_Sel_PreR_Probability"(w548) -> ()
      n478 = local write "LC_Sel_PreR_Tdelay"(w547) -> ()
      n479 = local write "LC_Sel_PreR_Count"(w546) -> ()
      n480 = local write "LC_Sel_PostR_OnOff"(w556) -> ()
      n481 = local write "LC_Sel_PostR_Block"(w544) -> ()
      n482 = local write "LC_Sel_PostR_Probability"(w543) -> ()
      n483 = local write "LC_Sel_PostR_Tdelay"(w542) -> ()
      n484 = local write "LC_Sel_PostR_Count"(w541) -> ()
      n485 = local write "LC_ENL_nRew1"(w396) -> ()
      n486 = local write "LC_ENL_nRew2"(w395) -> ()
      n487 = local write "LC_ENL2_nRew1"(w391) -> ()
      n488 = local write "LC_ENL2_nRew2"(w390) -> ()
      n489 = local write "LC_Cue_nRew1"(w383) -> ()
      n490 = local write "LC_Cue_nRew2"(w382) -> ()
      n491 = local write "LC_Cue2_nRew1"(w381) -> ()
      n492 = local write "LC_Cue2_nRew2"(w380) -> ()
      n493 = local write "LC_Sel_nRew1"(w379) -> ()
      n494 = local write "LC_Sel_nRew2"(w378) -> ()
    }
  }
  "output_dataLC" <- w4
  "output_dataExp" <- w1
